vi "MS Auto Operation.vi"() -> ()   [LabVIEW 2016]
uses:
  <vilib>/Analysis/Matrix/Datatypes/RealMatrix.ctl
  Subsystems/Global Variables.vi
  <vilib>/FPGAPlugInAG/PXI-7833R/niLvFpga_Open_PXI-7833R.vi
  <vilib>/Utility/error.llb/Error Cluster From Error Code.vi
  <vilib>/rvi/errors/niLvFpgaAdjustHostInterfaceError.vi
  <vilib>/FPGAPlugInAG/PXI-7833R/niLvFpga_Reset_PXI-7833R.vi
  <vilib>/FPGAPlugInAG/PXI-7833R/niLvFpga_Close_PXI-7833R.vi
  <vilib>/rvi/interface/nirviOpenFPGA/nirviOpenFPGA.xnode
  FPGA Bitfiles/PhantomControlPI_FPGATarget_QuadCtr2_E2412E44.lvbitx
  IRISS_FPGA_IO.vi
  <vilib>/rvi/interface/nirviReadWriteControl/nirviReadWriteControl.xnode
  <vilib>/rvi/interface/nirviMethod/nirviMethod.xnode
  <vilib>/rvi/interface/nirviCloseFPGA/nirviCloseFPGA.xnode
  Library/KevinLibraryAll/labview2011/kevLib2011.lvlib
  <vilib>/Analysis/Matrix/NI_Matrix.lvlib
  NiFpgaLv.dll
panel:
  out "Online Eye Model":T1
  in  "To Regulation":bool
  out "Trajectory Cluster":T2
  out "Eye Model Cluster":T4={"X Grid"=[], "Y Grid"=[], "Za_true Surf"=[], "Iris Center"=[], "Zp_true Surf"=[], "Pinv"=[[1.0, 0.0], [0.0, 1.0]], "za_true"=5.0, "za_work"=1.0, "zp_work"=-1.0, "zp_true"=-5.0}
  out "Update Mdl & Traj":bool=TRUE
  in  "Initialize":bool caption="To M/S"
  out "Stage PID Cluster":T5={"Stage Z PID"={"Kp"=0.0005, "Kd"=0.001, "Ki"=0.0}, "Stage Y PID"={"Kp"=0.0003, "Kd"=0.01, "Ki"=0.0}, "Stage X PID"={"Kp"=0.0003, "Kd"=0.01, "Ki"=0.0}}
  out "L1 to L4 PID Cluster":T6={"L1 PID Gains"={"Kp"=0.005, "Kd"=0.5, "Ki"=0.0005}, "L2 PID Gains"={"Kp"=0.01, "Kd"=1.0, "Ki"=0.0005}, "L3 PID Gains"={"Kp"=0.05, "Kd"=1.0, "Ki"=0.0005}, "L4 PID Gains"={"Kp"=0.1, "Kd"=1.0, "Ki"=0.0005}}
  in  "IRISS GUI":T7(tab)
  in  "Reroute Hold [sec]":dbl=10.0 caption="Hold [sec]"
  out "X Stage out [mm] 2":dbl caption="Stage X [mm]" format="%#.4f"
  out "Z Stage out [mm] 2":dbl caption="Stage Z [mm]" format="%#.4f"
  out "Y Stage out [mm] 2":dbl caption="Stage Y [mm]" format="%#.4f"
  out "Vacuum Force [mmHg]  2":i32 caption="[mmHg]"
  out "Next Speed":dbl=0.8 format="%#.2gx"
  out "Current Speed":dbl=0.2 format="%#_2gx"
  out "Next Depth":dbl=40.0 format="%#_g%%"
  out "Current Depth":dbl=20.0 format="%#_6g%%"
  in  "Depth Offset":dbl min=-30.0 max=70.0 step=5.0 format="%#_g%%"
  in  "Refractice Index":dbl=1.35
  in  "PO No-Fly":dbl=5.0 step=0.1 format="%#.2g"
  out "PO Cruising":dbl=5.0 format="%#.2g"
  in  "Iris Center":dbl=5.0 step=0.1 format="%#.2g"
  in  "AN Cruising":dbl=5.0 step=0.1 format="%#.2g"
  in  "AN No-Fly":dbl=5.0 step=0.1 format="%#.2g"
  in  "Iris XY Scaling":dbl[](array[numeric])=[1.0, 1.0] caption="Iris Scaling" min=0.5 max=2.0 step=0.05
  in  "Iris XY Center":dbl[](array[numeric])=[0.0, 5.0] caption="Iris Center" min=-5.0 max=5.0 step=0.25
  out "Asgn Pt Out of Bound":bool caption="Assign Pt OOB"
  out "Finished Late Counts":u16
  out "Emergency alarm":bool
  out "Remote sender engaged":bool
  in  "L2 PID Gains":cluster{"Kp":dbl, "Kd":dbl, "Ki":dbl}={"Kp"=0.01, "Kd"=1.0, "Ki"=0.005}
  in  "L3 PID Gains":cluster{"Kp":dbl, "Kd":dbl, "Ki":dbl}={"Kp"=0.05, "Kd"=1.0, "Ki"=0.0005}
  in  "L4 PID Gains":cluster{"Kp":dbl, "Kd":dbl, "Ki":dbl}={"Kp"=0.1, "Kd"=0.1, "Ki"=0.0005}
  in  "L1 PID Gains":cluster{"Kp":dbl, "Kd":dbl, "Ki":dbl}={"Kp"=0.01, "Kd"=0.5, "Ki"=0.001}
  out "Current System State":T8(ring)
  out "State changing":bool
  out "Current Run No.":u8
  out "No. of Runs":i32=5
  out "Tip out Posit":dbl[](array[numeric]) caption="Position [mm]" format="%#.3f"
  out "Tip cmd Posit":dbl[](array[numeric]) caption="Command [mm]" format="%#.3f"
  out "L4 out Posit":dbl caption="y [deg]" format="%#.2g"
  out "L4 cmd Posit":dbl caption="r [deg]" format="%#.2g"
  out "L3 out Posit":dbl caption="y [mm]" format="%#.2g"
  out "L3 cmd Posit":dbl caption="r [mm]" format="%#.2g"
  out "L2 out Posit":dbl caption="y [deg]" format="%#.2g"
  out "L2 cmd Posit":dbl caption="r [deg]" format="%#.2g"
  out "L1 out Posit":dbl caption="y [deg]" format="%#.2g"
  out "L1 cmd Posit":dbl caption="r [deg]" format="%#.2g"
  out "State Flag Array":bool[](array[boolean])
  in  "Speed Override":u16(ring)=3 items=["4x", "3x", "2x", "1x", "0.5x", "0.2x", "0.1x", "PAUSE"]
  out "Timer":i32 format="%<%M:%S>t"
  in  "Assign Point [mm]":dbl[](array[numeric])=[0.0, 5.0, 0.0]
  in  "Go to Assign Pt":bool
  out "Irrigation Engaged? 2":bool caption="Irrigation Engaged"
  in  "Clear Charts":bool
  out "AC Pressure [mmHg]":sgl
  out "Elaspsed Time":sgl
  in  "File Path":path=path "C:/KevData1.txt"
  in  "Take IOP Data":bool
  out "IOP File Exists":bool
  in  "Seconds of Data":sgl=5.0
  out "Period [ms]":i64=10
  in  "Irrigation?":bool
  in  "PID ON/OFF":bool
  in  "Vac PID Gains":cluster{"Kp":dbl, "Kd":dbl, "Ki":dbl, "Ts":dbl}={"Kp"=5.0, "Kd"=0.0, "Ki"=5.0, "Ts"=0.01}
  in  "Vac Cmd":sgl min=0 max=100 step=1 format="%#_13g"
  in  "Target IOP":sgl=20.0 min=0 max=100 step=1 format="%#_13g"
  out "IOP Ctrl":T9(graph)
  out "Pressure Sensors":T10(graph)
  in  "Remote Control Source":u16(ring) caption="Remote Source" items=["Surgical Console", "Joystick"]
  in  "Reset Joystick":bool caption="Encoder Reset"
  in  "Robot Command":dbl[](array[numeric])=[0.0, 0.0, 0.0, 0.0]
  out "OCT Z out [mm]":dbl caption="OCT Out Z [mm]" format="%#.4f"
  out "OCT Z cmd [mm]":dbl=6.0 caption="OCT Z Ref [mm]" min=0.0 max=12.0 step=0.5
  in  "OCT Z PID Gains":cluster{"Kp":dbl, "Kd":dbl, "Ki":dbl}={"Kp"=0.0003, "Kd"=0.0001, "Ki"=0.01}
  out "Z Stage out [mm]":dbl caption="Output Z [mm]" format="%#.4f"
  out "Z Stage cmd [mm]":dbl=6.0 caption="Reference Z [mm]" min=0.0 max=12.0 step=0.5
  out "Y Stage out [mm]":dbl caption="Output Y [mm]" format="%#.4f"
  out "Y Stage cmd [mm]":dbl=6.0 caption="Reference Y  [mm]" min=0.0 max=12.0 step=0.5
  out "X Stage out [mm]":dbl caption="Output X [mm]" format="%#.4f"
  out "X Stage cmd [mm]":dbl=6.0 caption="Reference X [mm]" min=0.0 max=12.0 step=0.5
  in  "Stage Z PID Gains":cluster{"Kp":dbl, "Kd":dbl, "Ki":dbl}={"Kp"=0.0005, "Kd"=0.001, "Ki"=0.0}
  in  "Stage Y PID Gains":cluster{"Kp":dbl, "Kd":dbl, "Ki":dbl}={"Kp"=0.0001, "Kd"=0.005, "Ki"=0.0}
  in  "Stage X PID Gains":cluster{"Kp":dbl, "Kd":dbl, "Ki":dbl}={"Kp"=0.0003, "Kd"=0.01, "Ki"=0.0}
  in  "Reroute Transit Vacf":dbl=100.0
  out "Irrigation Engaged?":bool
  in  "Z Rot Axis":dbl=1.0
  in  "Z Dist Thld":dbl[](array[numeric])=[0.5, 2.0] caption="Z Distance Threshould"
  in  "Vac Extremum":dbl[](array[numeric])=[80.0, 100.0] caption="Vacuum Extremum"
  out "Accurus Button":bool[](array[boolean]) caption="Remote Button Command"
  in  "Max Limit [mmHg]":dbl=600.0
  in  "Control: Vacuum Force":i8(slide) min=0 max=78 step=1 scale=0.0..78.0
  out "Voltage Output Ch. B":dbl(graph)
  out "Voltage Output Ch. A":dbl(graph)
  out "Accurus Engaged?":bool
  out "Vacuum Force [mmHg]":i32
  in  "Stop-and-Go":bool=TRUE
  in  "Min PC Gap":dbl=0.1 caption="Min PC Gap [mm]" min=0.0 max=10.0 step=0.1 format="%#.3g"
  in  "Min AC Gap":dbl=0.1 caption="Min AC Gap [mm]" min=0.0 max=10.0 step=0.1 format="%#.3g"
  out "Scaling":dbl[](array[numeric])=[1.0, 1.0, 1.0] caption="S" min=0.5 max=1.5 step=0.05 format="%#_3g"
  in  "Joint Limits":dbl[][](array[numeric])=[[-8.0, 35.0], [-35.0, 35.0], [-5.0, 10.0], [-180.0, 180.0]] format="%#.3g"
  out "First Trk Pt":dbl[](array[numeric]) format="%#.3g"
  in  "Offset Home 2 RCM":dbl[](array[numeric])=[-7.7, 37.0, 55.0, 0.0] format="%#.3g"
  out "Error(s) Out on Program End":errorcluster
  out "L4 Waveform Graph":dbl[](graph)
  out "L3 Waveform Graph":dbl[](graph)
  out "L2 Waveform Graph":dbl[](graph)
  out "L1 Waveform Graph":dbl[](graph)
  in  "Aiming Pt":dbl[](array[numeric])=[10.0, 0.0, -1.0, 0.0] format="%#.3g"
  in  "Engage Pt":dbl[](array[numeric])=[15.0, 0.0, 3.0, 0.0] format="%#.3g"
  in  "Rotation":dbl[](array[numeric])=[0.0, 0.0, 0.0] caption="R [deg]" min=-15.0 max=15.0 step=0.5 format="%#_3g"
  out "Translation":dbl[](array[numeric]) caption="T [mm]" min=-3.0 max=3.0 step=0.1 format="%#_3g"
  in  "Inc Ctrl":dbl[](array[numeric])=[0.1, 0.05, 0.05] caption="Increment Control"
  in  "Load Traj":bool caption="To M/S"
  in  "MS/Auto":bool
  in  "Retract":bool caption="To M/S"
  in  "Stop Accurus":bool caption="To M/S"
  in  "L3 Go Home":bool caption="To M/S"
  in  "Track":bool caption="To M/S"
  in  "Insert":bool caption="To M/S"
  in  "Program Stop":bool
  # "M/S\n\nAuto"
  # "Robot Status"
  # "Tool Tip Location"
  # "Tracking Planning"
  # "L1"
  # "X\nY\nZ"
  # "X\nY\nZ"
  # "L2"
  # "System Progress"
  # "Assign Point Rerouting"
  # "X\nY\nZ"
  # "L3"
  # "Homing finished"
  # "M/S initialization finished"
  # "Tool Cruising Boundaries"
  # "Trajecoty loading finished"
  # "XY-plane"
  # "Z-axis"
  # "Aiming finished"
  # "L4"
  # "Tool engaged"
  # "Tracking initialization finished"
  # "In Tracking"
  # "Rerouting finished"
  # "In regulation"
  # "Vacuum"
  # "X\nY"
  # "X\nY"
  # "L1"
  # "L2"
  # "L3"
  # "L4"
  # "Data Saving"
  # "IOP Feedback Control"
  # "XYZ Stage Control"
  # "OCT Z-Axis"
  # "Foot Pedal Buttons"
  # "Irrigation and Aspiration"
  # "Button 1"
  # "Button 2"
  # "Button 3"
  # "Rotation & Vacuum Force Scheduling"
  # "Joint Motion & Control"
  # "Calibration"
  # "Space Deform Parameters"
  # "L1"
  # "[deg]"
  # "S"
  # "L2"
  # "[deg]"
  # "R"
  # "[deg]"
  # "L3"
  # "[mm]"
  # "T"
  # "[mm]"
  # "L4"
  # "[deg]"
  # "First Track Point"
  # "AC & PC Gap"
  # "L1"
  # "[deg]"
  # "L2"
  # "[deg]"
  # "L3"
  # "[mm]"
  # "L4"
  # "[deg]"
  # "Error Message"
  # "Tracking Joint Limits"
  # "Incision"
  # "Min."
  # "Max."
  # "L1"
  # "L1"
  # "[deg]"
  # "L2"
  # "L2"
  # "[deg]"
  # "L3"
  # "L3"
  # "[mm]"
  # "L4"
  # "L4"
  # "[deg]"
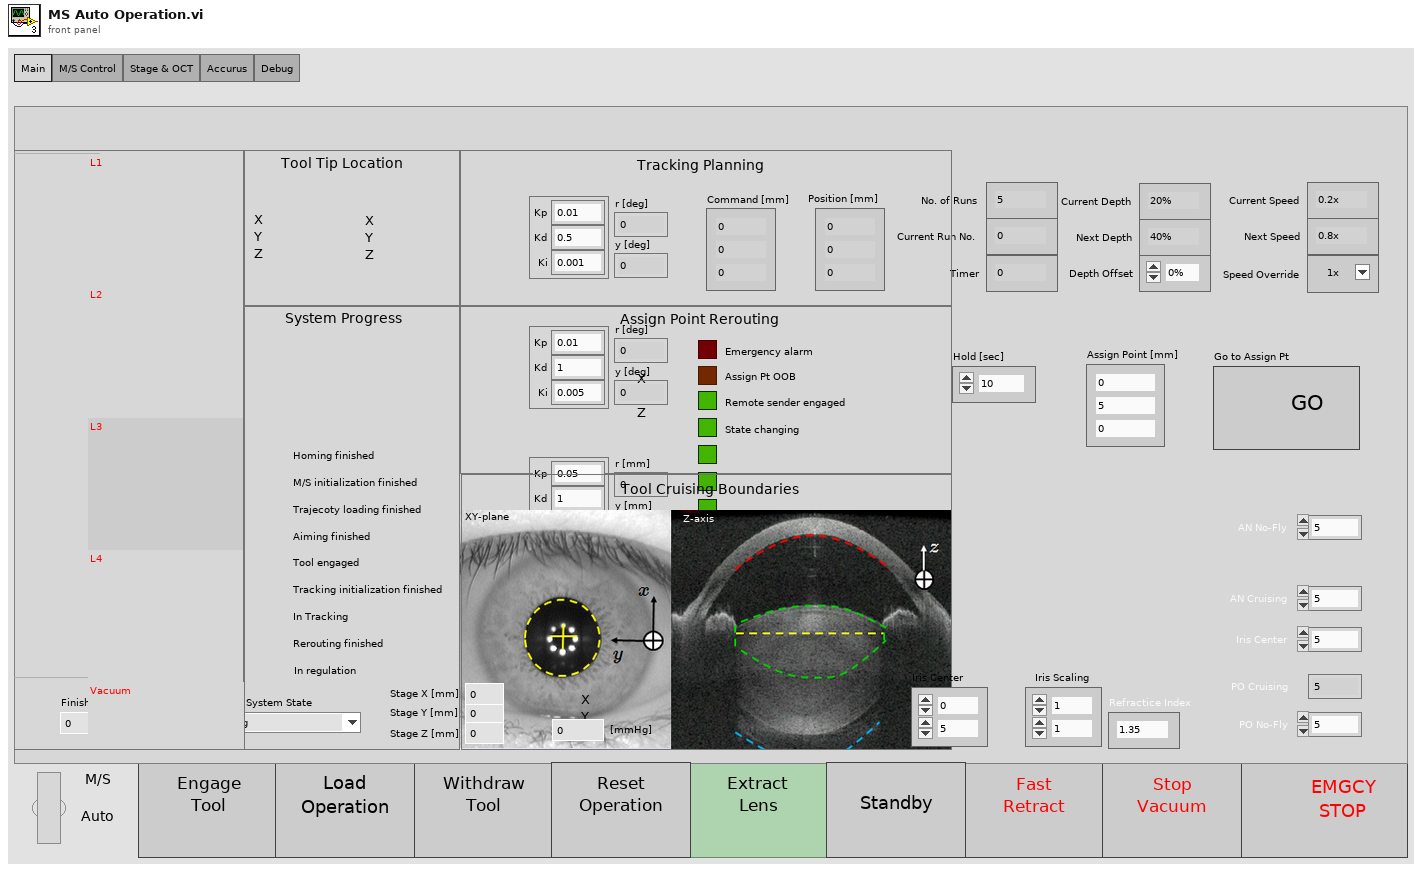
[diagram p1: front panel]
types:
  T1 = cluster{"za_true":dbl, "za_work":dbl, "zi":dbl, "zp_work":dbl, "zp_true":dbl, "Iris XY Center":dbl[], "Iris XY Scaling":dbl[]}
  T2 = cluster{"Traj Px Array":dbl[], "Traj Py Array":dbl[], "Traj Pz Array":dbl[], "Speed Array":dbl[], "Depth Array":dbl[]}
  T3 = typedef "NI_Matrix.lvlib/RealMatrix.ctl" = dbl[][]
  T4 = cluster{"X Grid":dbl[], "Y Grid":dbl[], "Za_true Surf":dbl[][], "Iris Center":dbl[], "Zp_true Surf":dbl[][], "Pinv":T3, "za_true":dbl, "za_work":dbl, "zp_work":dbl, "zp_true":dbl}
  T5 = cluster{"Stage Z PID":cluster{"Kp":dbl, "Kd":dbl, "Ki":dbl}, "Stage Y PID":cluster{"Kp":dbl, "Kd":dbl, "Ki":dbl}, "Stage X PID":cluster{"Kp":dbl, "Kd":dbl, "Ki":dbl}}
  T6 = cluster{"L1 PID Gains":cluster{"Kp":dbl, "Kd":dbl, "Ki":dbl}, "L2 PID Gains":cluster{"Kp":dbl, "Kd":dbl, "Ki":dbl}, "L3 PID Gains":cluster{"Kp":dbl, "Kd":dbl, "Ki":dbl}, "L4 PID Gains":cluster{"Kp":dbl, "Kd":dbl, "Ki":dbl}}
  T7 = enum32{"Main", "M/S Control", "Stage & OCT", "Accurus", "Debug"}
  T8 = enum16{"Homing", "M/S Initialization", "M/S Operation", "Aiming", "Engaging", "Trajectory Loading", "Tracking Initialization", "Tracking", "Rerouting", "Regulation"}
  T9 = cluster{"[0]":sgl, "[1]":sgl, "[2]":sgl, "[3]":sgl, "[4]":sgl, "[5]":sgl, "[6]":sgl, "[7]":sgl, "[8]":sgl}
  T10 = cluster{"pressure sensors[0]":sgl, "pressure sensors[1]":sgl, "pressure sensors[2]":sgl, "pressure sensors[3]":sgl, "pressure sensors[4]":sgl, "pressure sensors[5]":sgl, "pressure sensors[6]":sgl, "pressure sensors[7]":sgl, "pressure sensors[8]":sgl}
  T11 = cluster{"Prev L1 to L4 Posit":dbl[], "Prev Stage Posit":dbl[], "Prev OCT Z Posit":dbl}
  T12 = cluster{"L1 to L4 PID Cluster":cluster{"L1 PID Gains":cluster{"Kp":dbl, "Kd":dbl, "Ki":dbl}, "L2 PID Gains":cluster{"Kp":dbl, "Kd":dbl, "Ki":dbl}, "L3 PID Gains":cluster{"Kp":dbl, "Kd":dbl, "Ki":dbl}, "L4 PID Gains":cluster{"Kp":dbl, "Kd":dbl, "Ki":dbl}}, "Stage PID Cluster":cluster{"Stage Z PID":cluster{"Kp":dbl, "Kd":dbl, "Ki":dbl}, "Stage Y PID":cluster{"Kp":dbl, "Kd":dbl, "Ki":dbl}, "Stage X PID":cluster{"Kp":dbl, "Kd":dbl, "Ki":dbl}}, "OCT Z PID Gains":cluster{"Kp":dbl, "Kd":dbl, "Ki":dbl}}
  T13 = enum8{"Enabled", "Disabled", "Disabled and Grayed Out"}
  T14 = cluster{"Last L1 to L4 Posit":dbl[], "Last Stage Posit":dbl[], "Last OCT Z Posit":dbl}
  T15 = cluster{"za_true_0":dbl, "za_work_0":dbl, "zp_work_0":dbl, "zp_true_0":dbl, "IrisCenter_0":dbl[]}
  T16 = cluster{"X Grid":dbl[], "Y Grid":dbl[], "Za_true Surf":dbl[][], "Iris Center":dbl[], "Zp_true Surf":dbl[][], "Real Matrix":T3, "za_true":dbl, "za_work":dbl, "zp_work":dbl, "zp_true":dbl}
  T17 = cluster{"Accurus button":bool[], "Accurus engaged?":bool, "Vacuum Force":i32, "Accurus Ch. A Vout":dbl, "Accurus Ch. B Vout":dbl, "Irrigation engaged?":bool}
  T18 = cluster{"pressure sensors[0]":sgl, "pressure sensors[1]":sgl, "pressure sensors[2]":sgl, "pressure sensors[3]":sgl, "pressure sensors[4]":sgl, "pressure sensors[5]":sgl, "pressure sensors[6]":sgl, "pressure sensors[7]":sgl, "pressure sensors[8]":sgl}[]
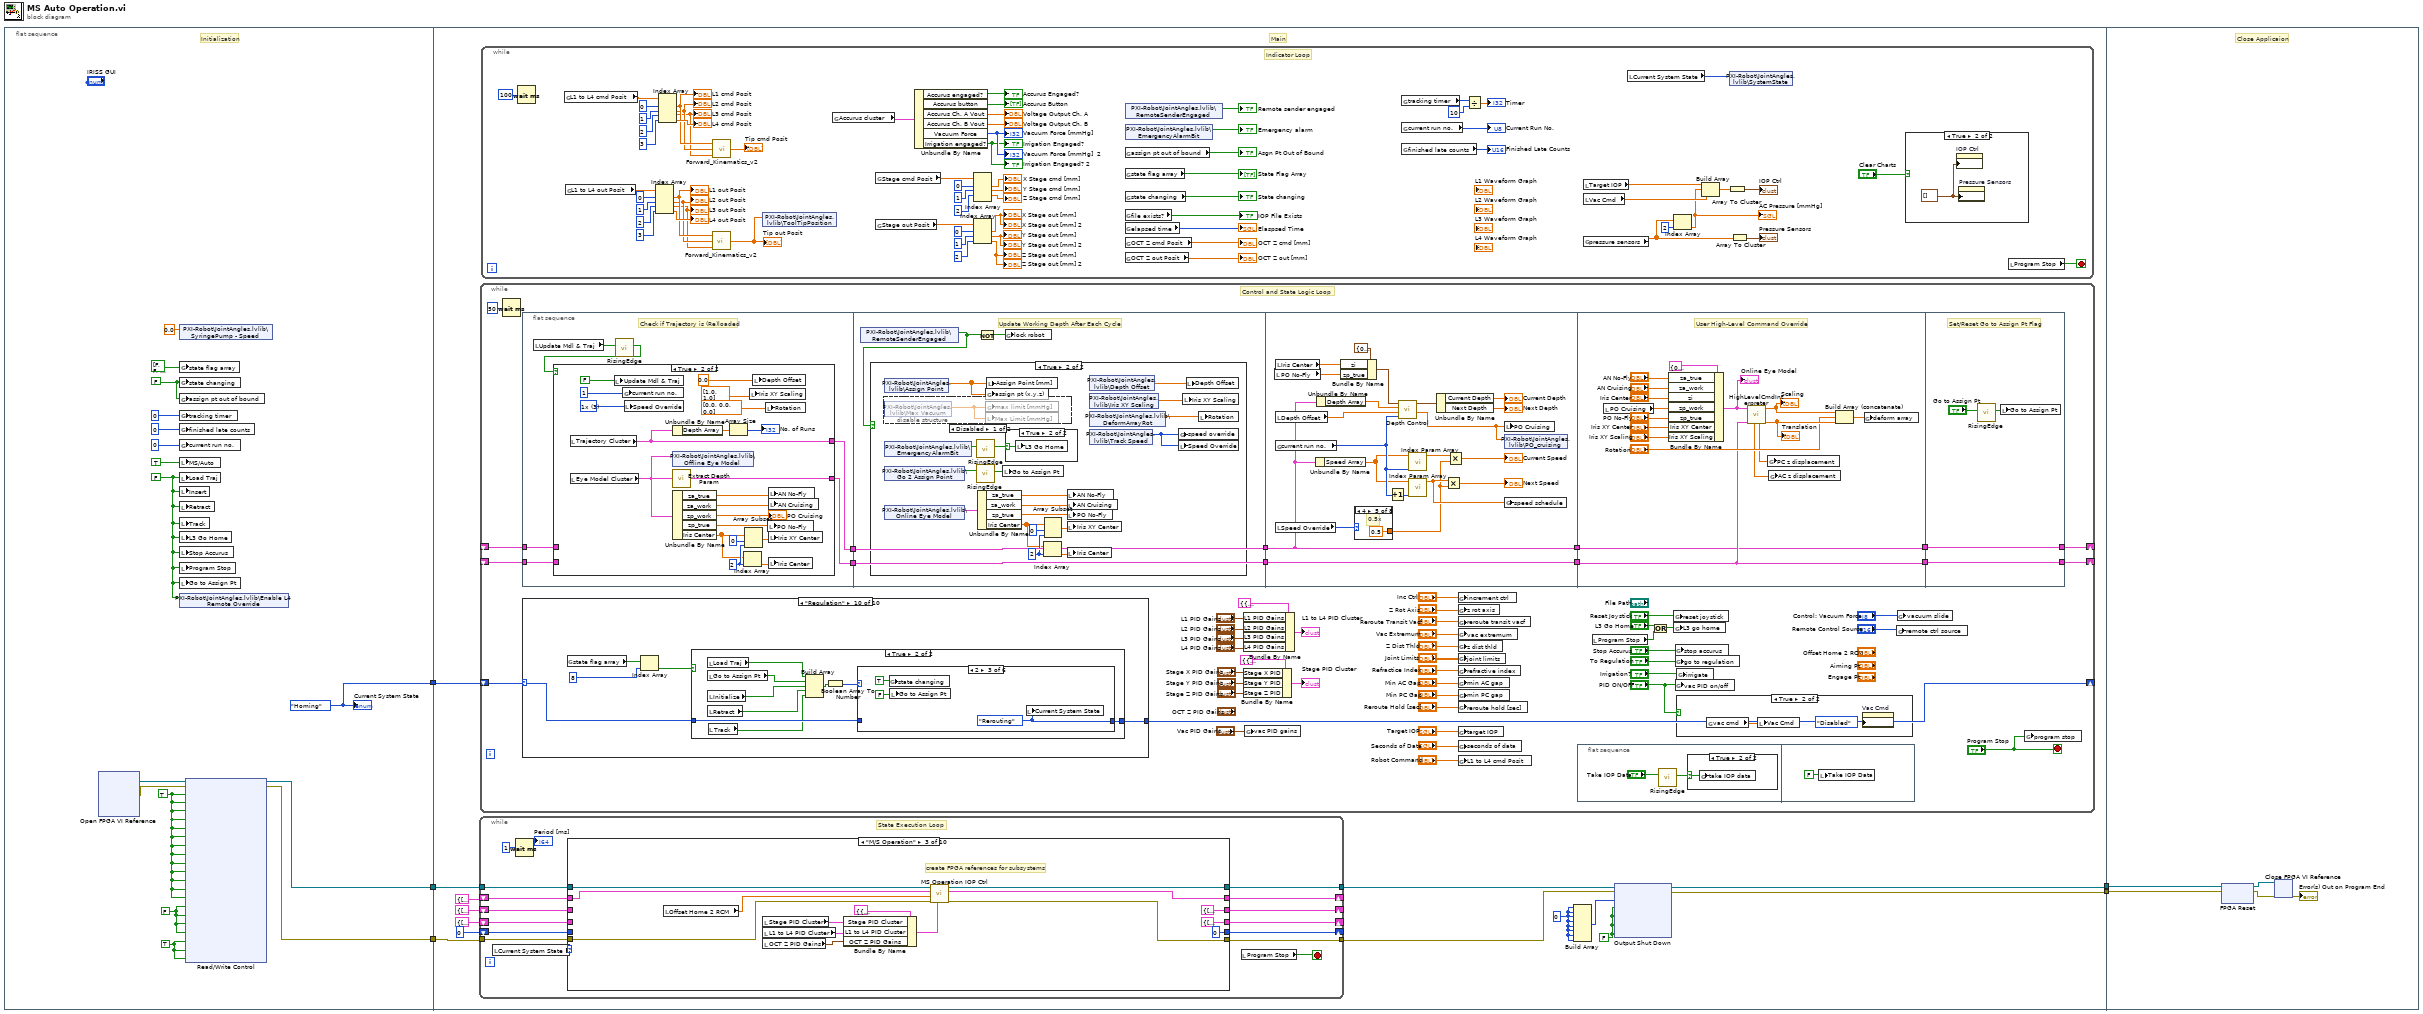
[diagram p0: block diagram]
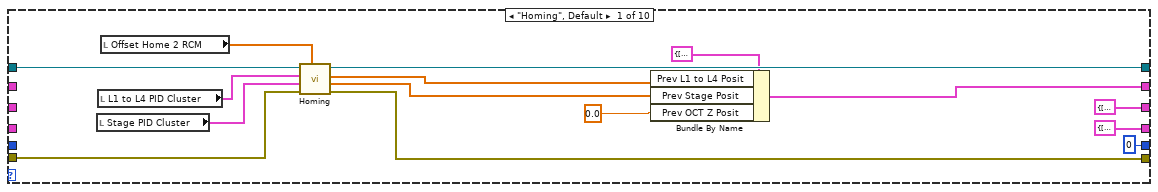
[diagram p3: hidden frame]
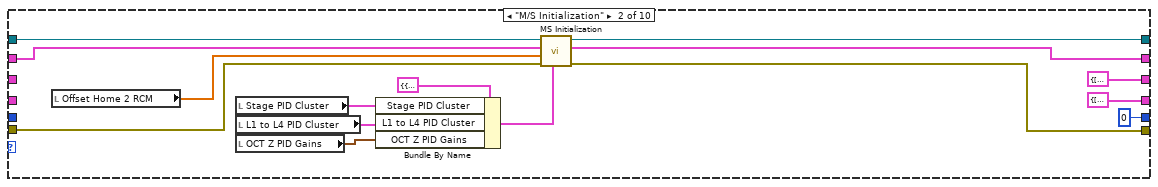
[diagram p4: hidden frame]
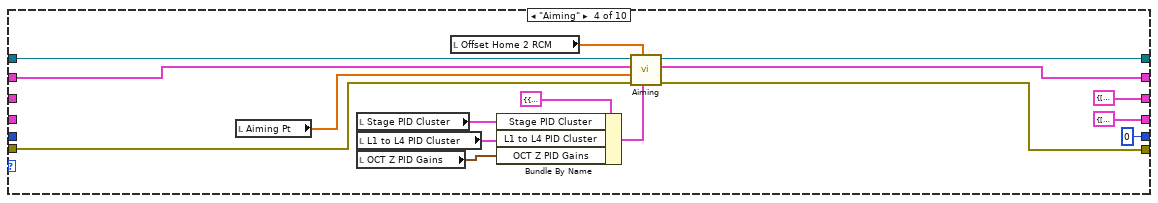
[diagram p5: hidden frame]
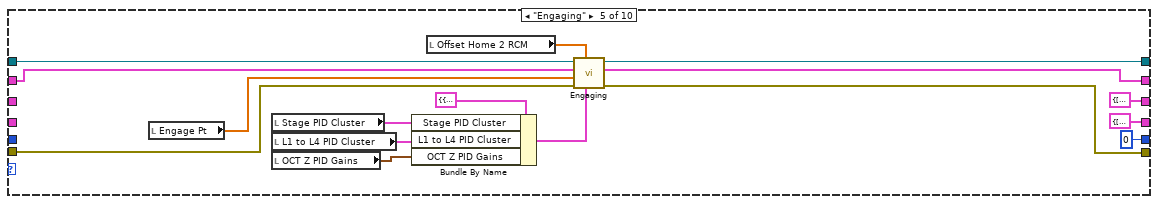
[diagram p6: hidden frame]
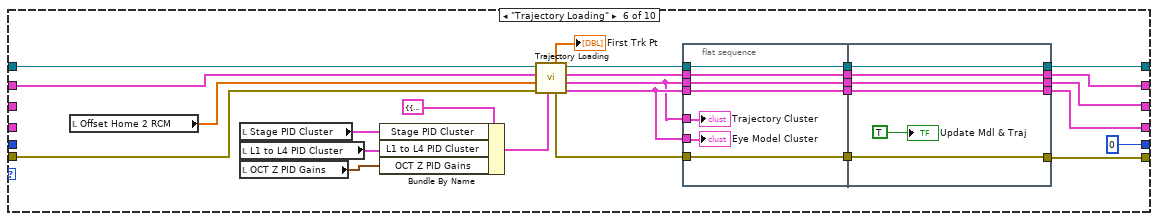
[diagram p7: hidden frame]
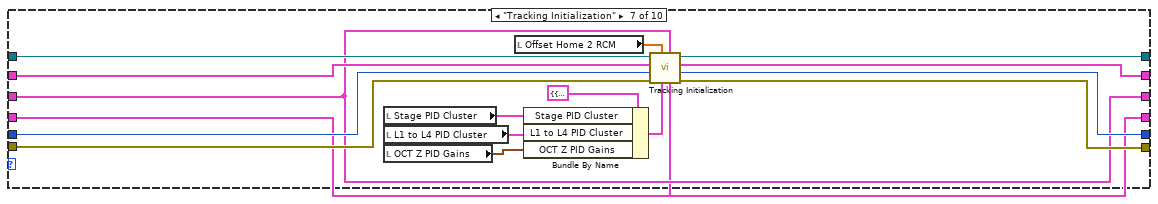
[diagram p8: hidden frame]
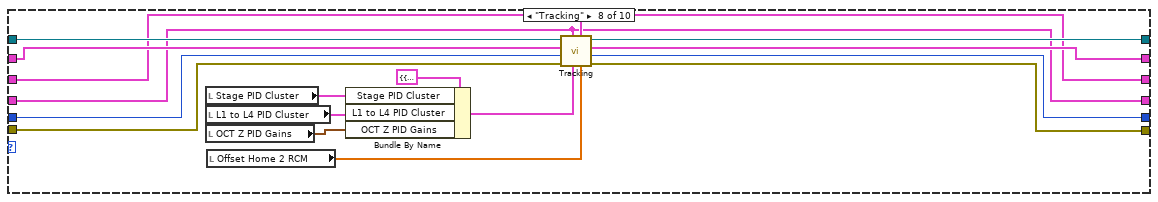
[diagram p9: hidden frame]
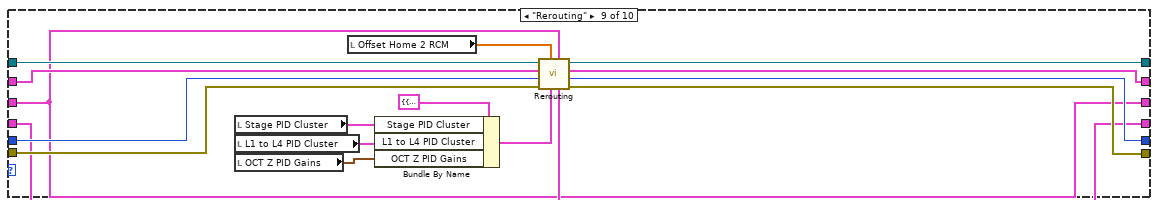
[diagram p10: hidden frame]
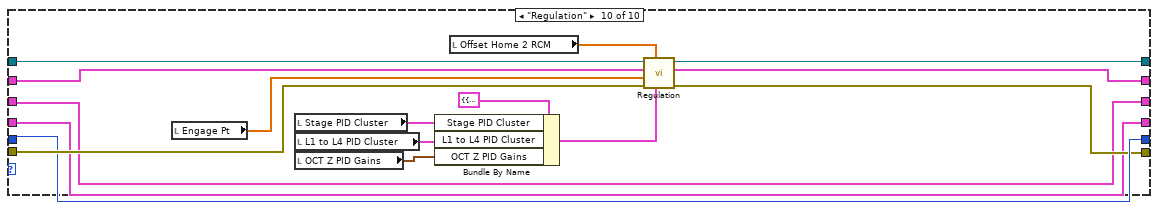
[diagram p11: hidden frame]
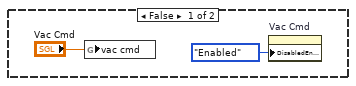
[diagram p13: hidden frame]
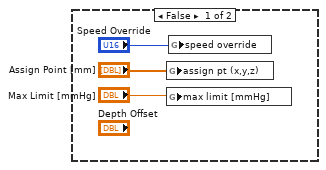
[diagram p15: hidden frame]
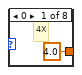
[diagram p18: hidden frame]
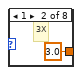
[diagram p19: hidden frame]
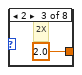
[diagram p20: hidden frame]
diagram:
  n1 = flat-sequence {
    tunnel: [w16] -> w5
    tunnel: [w15] -> w4
    tunnel: [w10] -> w3
    tunnel: w5 -> [w34]
    tunnel: w4 -> [w35]
    tunnel: w3 -> [w26]
    tunnel: [w28] -> w2
    tunnel: [w27] -> w1
    tunnel: w2 -> [w695]
    tunnel: w1 -> [w696]
    frame #0 {
      w10 = T8."Homing" ("Current State")
      w12 = FALSE ("state changing")
      w20 = TRUE ("Conn0/DIO12 Button 1")
      w19 = FALSE ("Reset")
      w21 = TRUE ("Reset")
      w13 = FALSE ("program stop")
      # "Initialization"
      n2 = xnode "Open FPGA VI Reference"() -> ("FPGA VI Reference Out"=w18:refnum<k20>, "error out"=w17:errorcluster)  [unwired: 2 in]
      n3 = shared-variable "PXI-Robot\\JointAngles.lvlib\\SyringePump - Speed"(0.0 ("SyringePump - Speed")) -> ()  [unwired: 1 in, 1 out]
      n4 = global write "Global Variables.vi" "state flag array"(bool[] [FALSE, FALSE, FALSE, FALSE, FALSE, FALSE, FALSE, FALSE, FALSE] ("state flag array")) -> ()
      n5 = global write "Global Variables.vi" "state changing"(w12) -> ()
      n6 = global write "Global Variables.vi" "assign pt out of bound"(w12) -> ()
      n7 = global write "Global Variables.vi" "tracking timer"(0 ("finished late counts")) -> ()
      n8 = global write "Global Variables.vi" "finished late counts"(u16 0 ("finished late counts")) -> ()
      n9 = global write "Global Variables.vi" "current run no."(u8 0 ("current run no.")) -> ()
      n10 = local write "MS/Auto"(TRUE ("MS/Auto")) -> ()
      n11 = local write "Load Traj"(w13) -> ()
      n12 = local write "Insert"(w13) -> ()
      n13 = local write "Retract"(w13) -> ()
      n14 = local write "Track"(w13) -> ()
      n15 = local write "L3 Go Home"(w13) -> ()
      n16 = local write "Stop Accurus"(w13) -> ()
      n17 = local write "Program Stop"(w13) -> ()
      n18 = local write "Go to Assign Pt"(w13) -> ()
      n19 = shared-variable "PXI-Robot\\JointAngles.lvlib\\Enable L4 Remote Override"(w13) -> ()  [unwired: 1 in, 1 out]
      n20 = xnode "Read/Write Control"("FPGA VI Reference In"=w18, "error in"=w17, "Reset 1"=w21, "Reset 3"=w21, "Reset 9"=w21, "Reset 10"=w21, "Reset 11"=w21, "Reset 12"=w21, "Reset 13"=w21, "Reset 14"=w21, "Reset 15"=w21, "Reset 16"=w21, "Reset 17"=w21, "Reset C1-1"=w21, "Reset C1-4"=w21, "INHB X"=w19, "INHB Y"=w19, "INHB Z"=w19, "INHB OCT Mot"=w19, "Conn0/DIO12 Button 1"=w20, "Conn0/DIO13 Button 2"=w20, "Conn0/DIO15 Button 4"=w20) -> ("FPGA VI Reference Out"=w15:refnum<k20>, "error out"=w16:errorcluster)
      "Current System State" <- w10
    }
    frame #1 {
      w32 = FALSE
      w24 = i16 0 ("element")
      # "Main"
      n21 = while {
        tunnel: w35 -> [w116]
        tunnel: w34 -> [w115]
        tunnel: [w114] -> w30
        tunnel: [w113] -> w29
        shift-right: [w111] -> _
        shift-left: T11 {"Prev L1 to L4 Posit"=[0.0, 0.0, 0.0, 0.0], "Prev Stage Posit"=[6.0, 6.0, 6.0], "Prev OCT Z Posit"=0.0} ("Prev Posit Cluster") -> [w112]
        shift-right: [w109] -> _
        shift-left: 0 -> [w108]
        shift-right: [w107] -> _
        shift-left: T2 {"Traj Px Array"=[], "Traj Py Array"=[], "Traj Pz Array"=[], "Speed Array"=[], "Depth Array"=[]} ("Trajectory Cluster") -> [w105]
        shift-right: [w106] -> _
        shift-left: T4 {"X Grid"=[], "Y Grid"=[], "Za_true Surf"=[], "Iris Center"=[0.0, 5.0, 0.0], "Zp_true Surf"=[], "Pinv"=[[1.0, 0.0], [0.0, 1.0]], "za_true"=0.0, "za_work"=0.0, "zp_work"=0.0, "zp_true"=0.0} ("Eye Model Cluster") -> [w104]
        stop <- w110 stop-if-true
        # "State Execution Loop"
        n22 = local read "Current System State"() -> (w117:T8)
        n23 = Wait (ms)(milliseconds to wait=u32 1) -> ()  [unwired: 1 out]
        n24 = case shown="\"M/S Operation\"" w117 {
          tunnel: w116 -> [w133 w148 w163 w177 w194 w221 w250 w266 w281 w293]
          tunnel: w115 -> [w132 w147 w162 w168 w186 w220 w249 w265 w275 w290]
          tunnel: [w131 w146 w161 w174 w195 w202 w248 w264 w282 w287] -> w114
          tunnel: [w130 w145 w160 w178 w183 w208 w247 w263 w269 w285] -> w113
          tunnel: w112 -> [_ w144 w159 w175 w184 w219 w245 w262 w274 w292]
          tunnel: [w129 w143 w158 w179 w192 w207 w246 w261 w272 w286] -> w111
          tunnel: [0 ("Last Index") 0 ("Last Index") 0 ("Last Index") 0 ("Last Index") 0 ("Last Index") 0 w237 w251 w270 w288] -> w109
          tunnel: w108 -> [_ _ _ _ _ _ w238 w252 w271 w288]
          tunnel: [T2 {"Traj Px Array"=[], "Traj Py Array"=[], "Traj Pz Array"=[], "Speed Array"=[], "Depth Array"=[]} ("Trajectory Cluster") T2 {"Traj Px Array"=[], "Traj Py Array"=[], "Traj Pz Array"=[], "Speed Array"=[], "Depth Array"=[]} ("Trajectory Cluster") T2 {"Traj Px Array"=[], "Traj Py Array"=[], "Traj Pz Array"=[], "Speed Array"=[], "Depth Array"=[]} ("Trajectory Cluster") T2 {"Traj Px Array"=[], "Traj Py Array"=[], "Traj Pz Array"=[], "Speed Array"=[], "Depth Array"=[]} ("Trajectory Cluster") T2 {"Traj Px Array"=[], "Traj Py Array"=[], "Traj Pz Array"=[], "Speed Array"=[], "Depth Array"=[]} ("Trajectory Cluster") w198 w236 w255 w267 w284] -> w107
          tunnel: [T4 {"X Grid"=[], "Y Grid"=[], "Za_true Surf"=[], "Iris Center"=[0.0, 5.0, 0.0], "Zp_true Surf"=[], "Pinv"=[[1.0, 0.0], [0.0, 1.0]], "za_true"=0.0, "za_work"=0.0, "zp_work"=0.0, "zp_true"=0.0} ("Eye Model Cluster") T4 {"X Grid"=[], "Y Grid"=[], "Za_true Surf"=[], "Iris Center"=[0.0, 5.0, 0.0], "Zp_true Surf"=[], "Pinv"=[[1.0, 0.0], [0.0, 1.0]], "za_true"=0.0, "za_work"=0.0, "zp_work"=0.0, "zp_true"=0.0} ("Eye Model Cluster") T4 {"X Grid"=[], "Y Grid"=[], "Za_true Surf"=[], "Iris Center"=[0.0, 5.0, 0.0], "Zp_true Surf"=[], "Pinv"=[[1.0, 0.0], [0.0, 1.0]], "za_true"=0.0, "za_work"=0.0, "zp_work"=0.0, "zp_true"=0.0} ("Eye Model Cluster") T4 {"X Grid"=[], "Y Grid"=[], "Za_true Surf"=[], "Iris Center"=[0.0, 5.0, 0.0], "Zp_true Surf"=[], "Pinv"=[[1.0, 0.0], [0.0, 1.0]], "za_true"=0.0, "za_work"=0.0, "zp_work"=0.0, "zp_true"=0.0} ("Eye Model Cluster") T4 {"X Grid"=[], "Y Grid"=[], "Za_true Surf"=[], "Iris Center"=[0.0, 5.0, 0.0], "Zp_true Surf"=[], "Pinv"=[[1.0, 0.0], [0.0, 1.0]], "za_true"=0.0, "za_work"=0.0, "zp_work"=0.0, "zp_true"=0.0} ("Eye Model Cluster") w197 w235 w254 w268 w283] -> w106
          tunnel: w105 -> [_ _ _ _ _ _ w236 w255 w267 w284]
          tunnel: w104 -> [_ _ _ _ _ _ w235 w254 w268 w283]
          frame "Homing", Default {
            n25 = local read "Stage PID Cluster"() -> (w125:T5)
            n26 = local read "L1 to L4 PID Cluster"() -> (w126:T6)
            n27 = local read "Offset Home 2 RCM"() -> (w128:dbl[])
            n28 = call "Homing.vi"("Offset Home 2 RCM"=w128, "error in"=w132, "Stage PID Cluster"=w125, "L1 to L4 PID Cluster"=w126, "FPGA VI Reference In"=w133) -> ("error out"=w130:errorcluster, "Last Stage Posit"=w122:dbl[], "Last L1 to L4 Posit"=w123:dbl[], "FPGA VI Reference Out"=w131:refnum<k20>)  [unwired: 3 in]
            n29 = Bundle By Name(cluster=T11 {"Prev L1 to L4 Posit"=[-0.5409, 0.04404050915429177, -1.917656453185038, 0.02068014705882353], "Prev Stage Posit"=[6.001471972029684, 5.996134588585126, 6.000298217087839], "Prev OCT Z Posit"=-0.0} ("Prev Posit Cluster"), "Prev L1 to L4 Posit"=w123, "Prev Stage Posit"=w122, "Prev OCT Z Posit"=0.0) -> (w129:T11)
          }
          frame "M/S Initialization" {
            n30 = local read "Offset Home 2 RCM"() -> (w137:dbl[])
            n31 = local read "Stage PID Cluster"() -> (w142:T5)
            n32 = local read "L1 to L4 PID Cluster"() -> (w141:T6)
            n33 = local read "OCT Z PID Gains"() -> (w140:cluster{"Kp":dbl, "Kd":dbl, "Ki":dbl})
            n34 = Bundle By Name(cluster=T12 {"L1 to L4 PID Cluster"={"L1 PID Gains"={"Kp"=0.005, "Kd"=0.5, "Ki"=0.0005}, "L2 PID Gains"={"Kp"=0.01, "Kd"=1.0, "Ki"=0.005}, "L3 PID Gains"={"Kp"=0.05, "Kd"=1.0, "Ki"=0.0005}, "L4 PID Gains"={"Kp"=0.1, "Kd"=0.1, "Ki"=0.0005}}, "Stage PID Cluster"={"Stage Z PID"={"Kp"=0.0005, "Kd"=0.001, "Ki"=0.0}, "Stage Y PID"={"Kp"=0.0003, "Kd"=0.01, "Ki"=0.0}, "Stage X PID"={"Kp"=0.0003, "Kd"=0.01, "Ki"=0.0}}, "OCT Z PID Gains"={"Kp"=0.0003, "Kd"=0.0001, "Ki"=0.01}} ("PID Cluster"), "Stage PID Cluster"=w142, "L1 to L4 PID Cluster"=w141, "OCT Z PID Gains"=w140) -> (w138:T12)
            n35 = call "MS Initialization.vi"("PID Cluster"=w138, "error in"=w147, "Offset Home 2 RCM"=w137, "Prev Posit Cluster"=w144, "FPGA VI Reference In"=w148) -> ("error out"=w145:errorcluster, "Last Posit Cluster"=w143:T14, "FPGA VI Reference Out"=w146:refnum<k20>)  [unwired: 4 in]
          }
          frame "M/S Operation" {
            # "create FPGA references for subsystems"
            n36 = local read "Offset Home 2 RCM"() -> (w152:dbl[])
            n37 = local read "Stage PID Cluster"() -> (w157:T5)
            n38 = local read "L1 to L4 PID Cluster"() -> (w156:T6)
            n39 = local read "OCT Z PID Gains"() -> (w155:cluster{"Kp":dbl, "Kd":dbl, "Ki":dbl})
            n40 = Bundle By Name(cluster=T12 {"L1 to L4 PID Cluster"={"L1 PID Gains"={"Kp"=0.005, "Kd"=0.5, "Ki"=0.0005}, "L2 PID Gains"={"Kp"=0.01, "Kd"=1.0, "Ki"=0.005}, "L3 PID Gains"={"Kp"=0.05, "Kd"=1.0, "Ki"=0.0005}, "L4 PID Gains"={"Kp"=0.1, "Kd"=0.1, "Ki"=0.0005}}, "Stage PID Cluster"={"Stage Z PID"={"Kp"=0.0005, "Kd"=0.001, "Ki"=0.0}, "Stage Y PID"={"Kp"=0.0003, "Kd"=0.01, "Ki"=0.0}, "Stage X PID"={"Kp"=0.0003, "Kd"=0.01, "Ki"=0.0}}, "OCT Z PID Gains"={"Kp"=0.0003, "Kd"=0.0001, "Ki"=0.01}} ("PID Cluster"), "Stage PID Cluster"=w157, "L1 to L4 PID Cluster"=w156, "OCT Z PID Gains"=w155) -> (w153:T12)
            n41 = call "MS Operation IOP Ctrl.vi"("PID Cluster"=w153, "error in"=w162, "Offset Home 2 RCM"=w152, "Prev Posit Cluster"=w159, "FPGA VI Reference In"=w163) -> ("error out"=w160:errorcluster, "Last Posit Cluster"=w158:T14, "FPGA VI Reference Out"=w161:refnum<k20>)  [unwired: 4 in]
          }
          frame "Aiming" {
            n42 = local read "Aiming Pt"() -> (w173:dbl[])
            n43 = local read "Stage PID Cluster"() -> (w172:T5)
            n44 = local read "L1 to L4 PID Cluster"() -> (w171:T6)
            n45 = local read "OCT Z PID Gains"() -> (w169:cluster{"Kp":dbl, "Kd":dbl, "Ki":dbl})
            n46 = local read "Offset Home 2 RCM"() -> (w176:dbl[])
            n47 = Bundle By Name(cluster=T12 {"L1 to L4 PID Cluster"={"L1 PID Gains"={"Kp"=0.005, "Kd"=0.5, "Ki"=0.0005}, "L2 PID Gains"={"Kp"=0.01, "Kd"=1.0, "Ki"=0.005}, "L3 PID Gains"={"Kp"=0.05, "Kd"=1.0, "Ki"=0.0005}, "L4 PID Gains"={"Kp"=0.1, "Kd"=0.1, "Ki"=0.0005}}, "Stage PID Cluster"={"Stage Z PID"={"Kp"=0.0005, "Kd"=0.001, "Ki"=0.0}, "Stage Y PID"={"Kp"=0.0003, "Kd"=0.01, "Ki"=0.0}, "Stage X PID"={"Kp"=0.0003, "Kd"=0.01, "Ki"=0.0}}, "OCT Z PID Gains"={"Kp"=0.0003, "Kd"=0.0001, "Ki"=0.01}} ("PID Cluster"), "Stage PID Cluster"=w172, "L1 to L4 PID Cluster"=w171, "OCT Z PID Gains"=w169) -> (w167:T12)
            n48 = call "Aiming.vi"("PID Cluster"=w167, "Offset Home 2 RCM"=w176, "error in"=w168, "Aiming Pt"=w173, "Prev Posit Cluster"=w175, "FPGA VI Reference In"=w177) -> ("error out"=w178:errorcluster, "Last Posit Cluster"=w179:T14, "FPGA VI Reference Out"=w174:refnum<k20>)  [unwired: 3 in]
          }
          frame "Engaging" {
            n49 = local read "Engage Pt"() -> (w185:dbl[])
            n50 = local read "Stage PID Cluster"() -> (w190:T5)
            n51 = local read "L1 to L4 PID Cluster"() -> (w189:T6)
            n52 = local read "OCT Z PID Gains"() -> (w188:cluster{"Kp":dbl, "Kd":dbl, "Ki":dbl})
            n53 = Bundle By Name(cluster=T12 {"L1 to L4 PID Cluster"={"L1 PID Gains"={"Kp"=0.005, "Kd"=0.5, "Ki"=0.0005}, "L2 PID Gains"={"Kp"=0.01, "Kd"=1.0, "Ki"=0.005}, "L3 PID Gains"={"Kp"=0.05, "Kd"=1.0, "Ki"=0.0005}, "L4 PID Gains"={"Kp"=0.1, "Kd"=0.1, "Ki"=0.0005}}, "Stage PID Cluster"={"Stage Z PID"={"Kp"=0.0005, "Kd"=0.001, "Ki"=0.0}, "Stage Y PID"={"Kp"=0.0003, "Kd"=0.01, "Ki"=0.0}, "Stage X PID"={"Kp"=0.0003, "Kd"=0.01, "Ki"=0.0}}, "OCT Z PID Gains"={"Kp"=0.0003, "Kd"=0.0001, "Ki"=0.01}} ("PID Cluster"), "Stage PID Cluster"=w190, "L1 to L4 PID Cluster"=w189, "OCT Z PID Gains"=w188) -> (w187:T12)
            n54 = local read "Offset Home 2 RCM"() -> (w193:dbl[])
            n55 = call "Engaging.vi"("PID Cluster"=w187, "Offset Home 2 RCM"=w193, "error in"=w186, "Engage Pt"=w185, "Prev Posit Cluster"=w184, "FPGA VI Reference In"=w194) -> ("error out"=w183:errorcluster, "Last Posit Cluster"=w192:T14, "FPGA VI Reference Out"=w195:refnum<k20>)  [unwired: 3 in]
          }
          frame "Trajectory Loading" {
            n56 = local read "Offset Home 2 RCM"() -> (w213:dbl[])
            n57 = local read "Stage PID Cluster"() -> (w218:T5)
            n58 = local read "L1 to L4 PID Cluster"() -> (w217:T6)
            n59 = local read "OCT Z PID Gains"() -> (w216:cluster{"Kp":dbl, "Kd":dbl, "Ki":dbl})
            n60 = Bundle By Name(cluster=T12 {"L1 to L4 PID Cluster"={"L1 PID Gains"={"Kp"=0.005, "Kd"=0.5, "Ki"=0.0005}, "L2 PID Gains"={"Kp"=0.01, "Kd"=1.0, "Ki"=0.005}, "L3 PID Gains"={"Kp"=0.05, "Kd"=1.0, "Ki"=0.0005}, "L4 PID Gains"={"Kp"=0.1, "Kd"=0.1, "Ki"=0.0005}}, "Stage PID Cluster"={"Stage Z PID"={"Kp"=0.0005, "Kd"=0.001, "Ki"=0.0}, "Stage Y PID"={"Kp"=0.0003, "Kd"=0.01, "Ki"=0.0}, "Stage X PID"={"Kp"=0.0003, "Kd"=0.01, "Ki"=0.0}}, "OCT Z PID Gains"={"Kp"=0.0003, "Kd"=0.0001, "Ki"=0.01}} ("PID Cluster"), "Stage PID Cluster"=w218, "L1 to L4 PID Cluster"=w217, "OCT Z PID Gains"=w216) -> (w214:T12)
            n61 = call "Trajectory Loading.vi"("PID Cluster"=w214, "error in"=w220, "Offset Home 2 RCM"=w213, "Prev Posit Cluster"=w219, "FPGA VI Reference In"=w221) -> ("Eye Model Cluster"=w200:T4, "Trajectory Cluster"=w196:T2, "Last Posit Cluster"=w206:T14, "FPGA VI Reference Out"=w204:refnum<k20>, "error out"=w210:errorcluster, "First Trk Pt"=→"First Trk Pt":dbl[])  [unwired: 1 in]
            n62 = flat-sequence {
              tunnel: w196 -> [w227]
              tunnel: w200 -> [w228]
              tunnel: w210 -> [w226]
              tunnel: [w226] -> w209
              tunnel: w206 -> [w225]
              tunnel: [w225] -> w205
              tunnel: w204 -> [w224]
              tunnel: [w224] -> w203
              tunnel: [w223] -> w201
              tunnel: w196 -> [w223]
              tunnel: w200 -> [w222]
              tunnel: [w222] -> w199
              tunnel: [w233] -> w208
              tunnel: w209 -> [w233]
              tunnel: [w232] -> w207
              tunnel: w205 -> [w232]
              tunnel: w203 -> [w231]
              tunnel: [w231] -> w202
              tunnel: w201 -> [w230]
              tunnel: w199 -> [w229]
              tunnel: [w230] -> w198
              tunnel: [w229] -> w197
              frame #0 {
                "Eye Model Cluster" <- w228
                "Trajectory Cluster" <- w227
              }
              frame #1 {
                "Update Mdl & Traj" <- TRUE
              }
            }
          }
          frame "Tracking Initialization" {
            n63 = local read "Stage PID Cluster"() -> (w243:T5)
            n64 = local read "L1 to L4 PID Cluster"() -> (w242:T6)
            n65 = local read "OCT Z PID Gains"() -> (w240:cluster{"Kp":dbl, "Kd":dbl, "Ki":dbl})
            n66 = local read "Offset Home 2 RCM"() -> (w244:dbl[])
            n67 = Bundle By Name(cluster=T12 {"L1 to L4 PID Cluster"={"L1 PID Gains"={"Kp"=0.005, "Kd"=0.5, "Ki"=0.0005}, "L2 PID Gains"={"Kp"=0.01, "Kd"=1.0, "Ki"=0.005}, "L3 PID Gains"={"Kp"=0.05, "Kd"=1.0, "Ki"=0.0005}, "L4 PID Gains"={"Kp"=0.1, "Kd"=0.1, "Ki"=0.0005}}, "Stage PID Cluster"={"Stage Z PID"={"Kp"=0.0005, "Kd"=0.001, "Ki"=0.0}, "Stage Y PID"={"Kp"=0.0003, "Kd"=0.01, "Ki"=0.0}, "Stage X PID"={"Kp"=0.0003, "Kd"=0.01, "Ki"=0.0}}, "OCT Z PID Gains"={"Kp"=0.0003, "Kd"=0.0001, "Ki"=0.01}} ("PID Cluster"), "Stage PID Cluster"=w243, "L1 to L4 PID Cluster"=w242, "OCT Z PID Gains"=w240) -> (w239:T12)
            n68 = call "Tracking Initialization.vi"("Eye Model Cluster"=w235, "Trajectory Cluster"=w236, "PID Cluster"=w239, "Offset Home 2 RCM"=w244, "error in"=w249, "Prev Index"=w238, "Prev Posit Cluster"=w245, "FPGA VI Reference In"=w250) -> ("error out"=w247:errorcluster, "Last Index"=w237:i32, "Last Posit Cluster"=w246:T14, "FPGA VI Reference Out"=w248:refnum<k20>)
          }
          frame "Tracking" {
            n69 = local read "Stage PID Cluster"() -> (w260:T5)
            n70 = local read "L1 to L4 PID Cluster"() -> (w259:T6)
            n71 = local read "OCT Z PID Gains"() -> (w258:cluster{"Kp":dbl, "Kd":dbl, "Ki":dbl})
            n72 = local read "Offset Home 2 RCM"() -> (w253:dbl[])
            n73 = Bundle By Name(cluster=T12 {"L1 to L4 PID Cluster"={"L1 PID Gains"={"Kp"=0.005, "Kd"=0.5, "Ki"=0.0005}, "L2 PID Gains"={"Kp"=0.01, "Kd"=1.0, "Ki"=0.005}, "L3 PID Gains"={"Kp"=0.05, "Kd"=1.0, "Ki"=0.0005}, "L4 PID Gains"={"Kp"=0.1, "Kd"=0.1, "Ki"=0.0005}}, "Stage PID Cluster"={"Stage Z PID"={"Kp"=0.0005, "Kd"=0.001, "Ki"=0.0}, "Stage Y PID"={"Kp"=0.0003, "Kd"=0.01, "Ki"=0.0}, "Stage X PID"={"Kp"=0.0003, "Kd"=0.01, "Ki"=0.0}}, "OCT Z PID Gains"={"Kp"=0.0003, "Kd"=0.0001, "Ki"=0.01}} ("PID Cluster"), "Stage PID Cluster"=w260, "L1 to L4 PID Cluster"=w259, "OCT Z PID Gains"=w258) -> (w256:T12)
            n74 = call "Tracking.vi"("Offset Home 2 RCM"=w253, "Trajectory Cluster"=w255, "PID Cluster"=w256, "Eye Model Cluster"=w254, "error in"=w265, "Resume Index"=w252, "Prev Posit Cluster"=w262, "FPGA VI Reference In"=w266) -> ("error out"=w263:errorcluster, "Leave Index"=w251:i32, "Last Posit Cluster"=w261:T14, "FPGA VI Reference Out"=w264:refnum<k20>)
          }
          frame "Rerouting" {
            n75 = local read "Stage PID Cluster"() -> (w279:T5)
            n76 = local read "L1 to L4 PID Cluster"() -> (w278:T6)
            n77 = local read "OCT Z PID Gains"() -> (w277:cluster{"Kp":dbl, "Kd":dbl, "Ki":dbl})
            n78 = local read "Offset Home 2 RCM"() -> (w273:dbl[])
            n79 = Bundle By Name(cluster=T12 {"L1 to L4 PID Cluster"={"L1 PID Gains"={"Kp"=0.005, "Kd"=0.5, "Ki"=0.0005}, "L2 PID Gains"={"Kp"=0.01, "Kd"=1.0, "Ki"=0.005}, "L3 PID Gains"={"Kp"=0.05, "Kd"=1.0, "Ki"=0.0005}, "L4 PID Gains"={"Kp"=0.1, "Kd"=0.1, "Ki"=0.0005}}, "Stage PID Cluster"={"Stage Z PID"={"Kp"=0.0005, "Kd"=0.001, "Ki"=0.0}, "Stage Y PID"={"Kp"=0.0003, "Kd"=0.01, "Ki"=0.0}, "Stage X PID"={"Kp"=0.0003, "Kd"=0.01, "Ki"=0.0}}, "OCT Z PID Gains"={"Kp"=0.0003, "Kd"=0.0001, "Ki"=0.01}} ("PID Cluster"), "Stage PID Cluster"=w279, "L1 to L4 PID Cluster"=w278, "OCT Z PID Gains"=w277) -> (w276:T12)
            n80 = call "Rerouting.vi"("Eye Model Cluster"=w268, "Trajectory Cluster"=w267, "PID Cluster"=w276, "Offset Home 2 RCM"=w273, "error in"=w275, "Prev Index"=w271, "Prev Posit Cluster"=w274, "FPGA VI Reference In"=w281) -> ("error out"=w269:errorcluster, "Last Index"=w270:i32, "Last Posit Cluster"=w272:T14, "FPGA VI Reference Out"=w282:refnum<k20>)
          }
          frame "Regulation" {
            n81 = local read "Engage Pt"() -> (w289:dbl[])
            n82 = local read "Stage PID Cluster"() -> (w297:T5)
            n83 = local read "L1 to L4 PID Cluster"() -> (w296:T6)
            n84 = local read "OCT Z PID Gains"() -> (w295:cluster{"Kp":dbl, "Kd":dbl, "Ki":dbl})
            n85 = Bundle By Name(cluster=T12 {"L1 to L4 PID Cluster"={"L1 PID Gains"={"Kp"=0.005, "Kd"=0.5, "Ki"=0.0005}, "L2 PID Gains"={"Kp"=0.01, "Kd"=1.0, "Ki"=0.005}, "L3 PID Gains"={"Kp"=0.05, "Kd"=1.0, "Ki"=0.0005}, "L4 PID Gains"={"Kp"=0.1, "Kd"=0.1, "Ki"=0.0005}}, "Stage PID Cluster"={"Stage Z PID"={"Kp"=0.0005, "Kd"=0.001, "Ki"=0.0}, "Stage Y PID"={"Kp"=0.0003, "Kd"=0.01, "Ki"=0.0}, "Stage X PID"={"Kp"=0.0003, "Kd"=0.01, "Ki"=0.0}}, "OCT Z PID Gains"={"Kp"=0.0003, "Kd"=0.0001, "Ki"=0.01}} ("PID Cluster"), "Stage PID Cluster"=w297, "L1 to L4 PID Cluster"=w296, "OCT Z PID Gains"=w295) -> (w291:T12)
            n86 = local read "Offset Home 2 RCM"() -> (w294:dbl[])
            n87 = call "Regulation.vi"("PID Cluster"=w291, "Offset Home 2 RCM"=w294, "error in"=w290, "Engage Pt"=w289, "Prev Posit Cluster"=w292, "FPGA VI Reference In"=w293) -> ("error out"=w285:errorcluster, "Last Posit Cluster"=w286:T14, "FPGA VI Reference Out"=w287:refnum<k20>)  [unwired: 3 in]
          }
        }
        n88 = local read "Program Stop"() -> (w110:bool)
      }
      n89 = while {
        shift-right: [w324] -> _
        shift-left: w26 -> [w325]
        shift-right: [w317] -> _
        shift-left: _ -> [w315]
        shift-right: [w316] -> _
        shift-left: _ -> [w314]
        stop <- "Program Stop" stop-if-true
        # "Control and State Logic Loop"
        n90 = Wait (ms)(milliseconds to wait=u32 50) -> ()  [unwired: 1 out]
        n91 = flat-sequence {
          tunnel: [w361] -> w321
          tunnel: [w360] -> w320
          tunnel: w315 -> [w359]
          tunnel: w314 -> [w358]
          tunnel: w321 -> [w389]
          tunnel: w320 -> [w388]
          tunnel: [w389] -> w310
          tunnel: [w388] -> w308
          tunnel: w310 -> [w416]
          tunnel: [w416] -> w309
          tunnel: w308 -> [w433]
          tunnel: [w433] -> w307
          tunnel: [w453] -> w319
          tunnel: w309 -> [w451]
          tunnel: [w451] -> w318
          tunnel: w307 -> [w453]
          tunnel: [w460] -> w316
          tunnel: w319 -> [w460]
          tunnel: [w459] -> w317
          tunnel: w318 -> [w459]
          frame #0 {
            # "Check if Trajectory is (Re)loaded"
            n92 = local read "Update Mdl & Traj"() -> (w363:bool)
            n93 = call "RisingEdge.vi"("Signal In"=w363) -> ("Rising Edge"=w362:bool)  [unwired: 10 in]
            n94 = case shown="True" w362 {
              tunnel: [w364 w385] -> w360
              tunnel: [w365 w374] -> w361
              tunnel: w359 -> [w365 _]
              tunnel: w358 -> [w364 _]
              frame False {
                # "Use Nominal Model & Trajectory"
              }
              frame True {
                w367 = u16 3 items=["4x", "3x", "2x", "1x", "0.5x", "0.2x", "0.1x", "PAUSE"] ("Speed Override")
                w379 = 2 ("index")
                # "Update Trajectory and Model after \"Trajectory Loading\""
                n95 = local read "Trajectory Cluster"() -> (w374:T2)
                n96 = local read "Eye Model Cluster"() -> (w372:T4)
                n97 = local write "Update Mdl & Traj"(FALSE ("Update Model")) -> ()
                n98 = global write "Global Variables.vi" "current run no."(u8 1 ("current run no.")) -> ()
                n99 = local write "Speed Override"(w367) -> ()
                n100 = Unbundle By Name(w374) -> ("Depth Array"=w376:dbl[])
                n101 = shared-variable "PXI-Robot\\JointAngles.lvlib\\Offline Eye Model"(w372) -> ()  [unwired: 1 in, 1 out]
                n102 = call "Extract Depth Param.vi"("Eye Model Cluster"=w372) -> ("Nominal Model param"=w385:T15)
                n103 = Unbundle By Name(w372) -> ("za_true"=w384:dbl, "za_work"=w383:dbl, "zp_work"=→"PO Cruising":dbl, "zp_true"=w381:dbl, "Iris Center"=w378:dbl[])
                n104 = Array Size(array=w376) -> (size(s)=→"No. of Runs":i32)
                n105 = Index Array(array=w378, index=w379) -> (element=w382:dbl)
                n106 = Array Subset(array=w378, index=0, length=w379) -> (w377:dbl[])
                n107 = local write "Iris XY Scaling"(dbl[] [1.0, 1.0]) -> ()
                n108 = local write "Depth Offset"(0.0 ("Depth Offset")) -> ()
                n109 = local write "Rotation"(dbl[] [0.0, 0.0, 0.0]) -> ()
                n110 = local write "PO No-Fly"(w381) -> ()
                n111 = local write "AN No-Fly"(w384) -> ()
                n112 = local write "AN Cruising"(w383) -> ()
                n113 = local write "Iris XY Center"(w377) -> ()
                n114 = local write "Iris Center"(w382) -> ()
              }
            }
          }
          frame #1 {
            # "Update Working Depth After Each Cycle"
            n115 = shared-variable "PXI-Robot\\JointAngles.lvlib\\RemoteSenderEngaged"() -> (w386:bool)  [unwired: 1 in, 1 out]
            n116 = case shown="True" w386 {
              frame False {
                n117 = global write "Global Variables.vi" "assign pt (x,y,z)"("Assign Point [mm]") -> ()
                n118 = global write "Global Variables.vi" "max limit [mmHg]"("Max Limit [mmHg]") -> ()
                n119 = global write "Global Variables.vi" "speed override"("Speed Override") -> ()
              }
              frame True {
                w396 = 2 ("index")
                n120 = disable-structure shown="Disabled" {
                  frame Disabled {
                    n121 = shared-variable "PXI-Robot\\JointAngles.lvlib\\Max Vacuum"() -> (w411:dbl)  [unwired: 1 in, 1 out]
                    n122 = global write "Global Variables.vi" "max limit [mmHg]"(w411) -> ()
                    n123 = local write "Max Limit [mmHg]"(w411) -> ()
                  }
                  frame Enabled {
                  }
                }
                n124 = shared-variable "PXI-Robot\\JointAngles.lvlib\\Assign Point"() -> (w409:dbl[])  [unwired: 1 in, 1 out]
                n125 = shared-variable "PXI-Robot\\JointAngles.lvlib\\EmergencyAlarmBit"() -> (w408:bool)  [unwired: 1 in, 1 out]
                n126 = shared-variable "PXI-Robot\\JointAngles.lvlib\\Go 2 Assign Point"() -> (w405:bool)  [unwired: 1 in, 1 out]
                n127 = shared-variable "PXI-Robot\\JointAngles.lvlib\\Online Eye Model"() -> (w401:T16)  [unwired: 1 in, 1 out]
                n128 = call "RisingEdge.vi"("Signal In"=w405) -> ("Rising Edge"=w406:bool)  [unwired: 10 in]
                n129 = call "RisingEdge.vi"("Signal In"=w408) -> ("Rising Edge"=w407:bool)  [unwired: 10 in]
                n130 = Unbundle By Name(w401) -> ("za_true"=w404:dbl, "za_work"=w403:dbl, "zp_true"=w402:dbl, "Iris Center"=w393:dbl[])
                n131 = global write "Global Variables.vi" "assign pt (x,y,z)"(w409) -> ()
                n132 = local write "Assign Point [mm]"(w409) -> ()
                n133 = local write "Go to Assign Pt"(w406) -> ()
                n134 = case shown="True" w407 {
                  selector: w407 -> [_ w412]
                  frame False {
                  }
                  frame True {
                    n135 = local write "L3 Go Home"(w412) -> ()
                  }
                }
                n136 = Index Array(array=w393, index=w396) -> (element=w394:dbl)
                n137 = Array Subset(array=w393, index=0, length=w396) -> (w397:dbl[])
                n138 = local write "AN No-Fly"(w404) -> ()
                n139 = local write "AN Cruising"(w403) -> ()
                n140 = local write "PO No-Fly"(w402) -> ()
                n141 = local write "Iris XY Center"(w397) -> ()
                n142 = local write "Iris Center"(w394) -> ()
                n143 = shared-variable "PXI-Robot\\JointAngles.lvlib\\Depth Offset"() -> (w400:dbl)  [unwired: 1 in, 1 out]
                n144 = shared-variable "PXI-Robot\\JointAngles.lvlib\\Iris XY Scaling"() -> (w399:dbl[])  [unwired: 1 in, 1 out]
                n145 = shared-variable "PXI-Robot\\JointAngles.lvlib\\DeformArrayRot"() -> (w398:dbl[])  [unwired: 1 in, 1 out]
                n146 = shared-variable "PXI-Robot\\JointAngles.lvlib\\Track Speed"() -> (w410:u16)  [unwired: 1 in, 1 out]
                n147 = global write "Global Variables.vi" "speed override"(w410) -> ()
                n148 = local write "Speed Override"(w410) -> ()
                n149 = local write "Iris XY Scaling"(w399) -> ()
                n150 = local write "Depth Offset"(w400) -> ()
                n151 = local write "Rotation"(w398) -> ()
              }
            }
            n152 = Not(x=w386) -> (.not. x?=w387:bool)
            n153 = global write "Global Variables.vi" "lock robot"(w387) -> ()
          }
          frame #2 {
            n154 = local read "PO No-Fly"() -> (w427:dbl)
            n155 = local read "Iris Center"() -> (w428:dbl)
            n156 = local read "Depth Offset"() -> (w432:dbl)
            n157 = global read "Global Variables.vi" "current run no."() -> (w425:u8)
            n158 = local read "Speed Override"() -> (w422:u16)
            n159 = Unbundle By Name(w416) -> ("Speed Array"=w424:dbl[])
            n160 = Unbundle By Name(w416) -> ("Depth Array"=w423:dbl[])
            n161 = Bundle By Name(cluster=cluster{"zi":dbl, "zp_true":dbl} {"zi"=0.0, "zp_true"=-2.5} ("z Cluster"), "zi"=w428, "zp_true"=w427) -> (w414:cluster{"zi":dbl, "zp_true":dbl})
            n162 = case shown="4" w422 {
              tunnel: [4.0 ("y") 3.0 ("y") 2.0 ("y") 1.0 ("y") 0.5 ("y") 0.2 ("y") 0.1 ("y") 0.0 ("y")] -> w419
              frame 0 {
                # "4X"
              }
              frame 1 {
                # "3X"
              }
              frame 2 {
                # "2X"
              }
              frame 3, Default {
                # "1x"
              }
              frame 4 {
                # "0.5x"
              }
              frame 5 {
                # "0.2x"
              }
              frame 6 {
                # "0.1x"
              }
              frame 7 {
                # "Pause"
              }
            }
            n163 = Increment(x=w425) -> (x+1=w426:u8)
            n164 = call "Depth Control.vi"("Current Run No."=w425, "Depth Offset"=w432, "Depth Array"=w423, "z Cluster"=w414) -> ("zp_work"=w413:dbl, "Schedule Depth & Speed"=w431:cluster{"Next Depth":dbl, "Current Depth":dbl})  [unwired: 6 in]
            n165 = call "Index Param Array.vi"("Index"=w425, "Array Input"=w424) -> ("Index Output"=w420:dbl)  [unwired: 9 in]
            n166 = call "Index Param Array.vi"("Index"=w426, "Array Input"=w424) -> ("Index Output"=w421:dbl)  [unwired: 9 in]
            n167 = Unbundle By Name(w431) -> ("Current Depth"=→"Current Depth":dbl, "Next Depth"=→"Next Depth":dbl)
            n168 = Multiply(x=w421, y=w419) -> (x*y=→"Next Speed":dbl)
            n169 = Multiply(x=w420, y=w419) -> (x*y=→"Current Speed":dbl)
            n170 = local write "PO Cruising"(w413) -> ()
            n171 = shared-variable "PXI-Robot\\JointAngles.lvlib\\PO_cruising"(w413) -> ()  [unwired: 1 in, 1 out]
            n172 = global write "Global Variables.vi" "speed schedule"(w421) -> ()
          }
          frame #3 {
            # "User High-Level Command Override"
            n173 = local read "PO Cruising"() -> (w442:dbl)
            n174 = Bundle By Name(cluster=T1 {"za_true"=0.0, "za_work"=0.0, "zi"=0.0, "zp_work"=0.0, "zp_true"=0.0, "Iris XY Center"=[0.0, 5.0], "Iris XY Scaling"=[1.0, 1.0]} ("High Level cmd"), "za_true"="AN No-Fly", "za_work"="AN Cruising", "zi"="Iris Center", "zp_work"=w442, "zp_true"="PO No-Fly", "Iris XY Center"="Iris XY Center", "Iris XY Scaling"="Iris XY Scaling") -> (w452:T1)
            "Online Eye Model" <- w452
            n175 = call "HighLevelCmdInterpreter.vi"("Nominal Model param"=w453, "High Level cmd"=w452) -> ("Translation Array"=w457:dbl[], "Scaling Array"=w458:dbl[], "PC Displacement"=w454:dbl, "AC Displacement"=w450:dbl)  [unwired: 6 in]
            "Scaling" <- w458
            "Translation" <- w457
            n176 = global write "Global Variables.vi" "PC z displacement"(w454) -> ()
            n177 = global write "Global Variables.vi" "AC z displacement"(w450) -> ()
            n178 = Build Array (concatenate)(w458, "Rotation", w457) -> (w455:dbl[])
            n179 = global write "Global Variables.vi" "deform array"(w455) -> ()
          }
          frame #4 {
            # "Set/Reset Go to Assign Pt Flag"
            n180 = call "RisingEdge.vi"("Signal In"="Go to Assign Pt") -> ("Rising Edge"=w462:bool)  [unwired: 10 in]
            n181 = local write "Go to Assign Pt"(w462) -> ()
          }
        }
        n182 = case shown="\"Regulation\"" w325 {
          selector: w325 -> [w465 w471 w487 w498 w517 w542 w550 w580 w618 w645]
          tunnel: [w464 w472 w486 w497 w518 w543 w551 w581 w619 w646] -> w324
          frame "Homing", Default {
            n183 = global read "Global Variables.vi" "state flag array"() -> (w466:bool[])
            n184 = Index Array(array=w466, index=0) -> (element=w463:bool)
            n185 = case shown="False" w463 {
              tunnel: [w468 w469] -> w464
              tunnel: w465 -> [w468 _]
              frame False {
                # "homing in process"
              }
              frame True {
                w469 = T8."M/S Initialization" ("Current State")
                # "finish homing"
                n186 = global write "Global Variables.vi" "state changing"(TRUE ("state changing")) -> ()
                n187 = local write "Current System State"(w469) -> ()
              }
            }
          }
          frame "M/S Initialization" {
            n188 = global read "Global Variables.vi" "state flag array"() -> (w474:bool[])
            n189 = Index Array(array=w474, index=1) -> (element=w473:bool)
            n190 = case shown="False" w473 {
              tunnel: [w476 w478] -> w472
              tunnel: w471 -> [w476 _]
              frame False {
                n191 = property on="MS/Auto" class="Bool (strict)"("DisabledEnum"=T13."Disabled and Grayed Out" ("Disabled")) -> ()  [unwired: 2 in, 2 out]
              }
              frame True {
                w478 = T8."M/S Operation" ("Current State")
                n192 = global write "Global Variables.vi" "state changing"(TRUE ("state changing")) -> ()
                n193 = property on="MS/Auto" class="Bool (strict)"("DisabledEnum"=T13."Enabled" ("Disabled")) -> ()  [unwired: 2 in, 2 out]
                n194 = local write "Current System State"(w478) -> ()
              }
            }
          }
          frame "M/S Operation" {
            n195 = local read "Load Traj"() -> (w483:bool)
            n196 = local read "MS/Auto"() -> (w485:bool)
            n197 = Not(x=w485) -> (.not. x?=w484:bool)
            n198 = Build Array(w484, w483) -> (w482:bool[])
            n199 = Boolean Array To Number(Boolean array=w482) -> (number=w481:u32)
            n200 = case shown="2" w481 {
              tunnel: w487 -> [w488 _ _]
              tunnel: [w488 w491 w494] -> w486
              frame 0, Default {
              }
              frame 1 {
                w491 = T8."Aiming" ("Current State")
                n201 = global write "Global Variables.vi" "state changing"(TRUE ("state changing")) -> ()
                n202 = property on="MS/Auto" class="Bool (strict)"("DisabledEnum"=T13."Disabled and Grayed Out" ("Disabled")) -> ()  [unwired: 2 in, 2 out]
                n203 = local write "Current System State"(w491) -> ()
              }
              frame 2 {
                w494 = T8."Trajectory Loading" ("Current State")
                n204 = global write "Global Variables.vi" "state changing"(TRUE ("state changing")) -> ()
                n205 = local write "Load Traj"(FALSE ("Load Traj")) -> ()
                n206 = property on="MS/Auto" class="Bool (strict)"("DisabledEnum"=T13."Disabled and Grayed Out" ("Disabled")) -> ()  [unwired: 2 in, 2 out]
                n207 = local write "MS/Auto"(FALSE ("MS/Auto")) -> ()
                n208 = local write "Current System State"(w494) -> ()
              }
            }
          }
          frame "Aiming" {
            n209 = global read "Global Variables.vi" "state flag array"() -> (w500:bool[])
            n210 = Index Array(array=w500, index=3) -> (element=w499:bool)
            n211 = case shown="True" w499 {
              tunnel: w498 -> [w502 w505]
              tunnel: [w502 w504] -> w497
              frame False {
              }
              frame True {
                n212 = property on="MS/Auto" class="Bool (strict)"("DisabledEnum"=T13."Enabled" ("Disabled")) -> ()  [unwired: 2 in, 2 out]
                n213 = Build Array("Insert", "MS/Auto") -> (w509:bool[])
                n214 = Boolean Array To Number(Boolean array=w509) -> (number=w506:u32)
                n215 = case shown="0, Default" w506 {
                  tunnel: w505 -> [w510 _ _]
                  tunnel: [w510 w512 w515] -> w504
                  frame 0, Default {
                  }
                  frame 1 {
                    w512 = T8."Engaging" ("Current State")
                    n216 = global write "Global Variables.vi" "state changing"(TRUE ("state changing")) -> ()
                    n217 = local write "Insert"(FALSE ("Enter")) -> ()
                    n218 = property on="MS/Auto" class="Bool (strict)"("DisabledEnum"=T13."Disabled and Grayed Out" ("Disabled")) -> ()  [unwired: 2 in, 2 out]
                    n219 = local write "Current System State"(w512) -> ()
                  }
                  frame 2 {
                    w515 = T8."M/S Initialization" ("Current State")
                    n220 = global write "Global Variables.vi" "state changing"(TRUE ("state changing")) -> ()
                    n221 = local write "Current System State"(w515) -> ()
                  }
                }
              }
            }
          }
          frame "Engaging" {
            n222 = global read "Global Variables.vi" "state flag array"() -> (w520:bool[])
            n223 = Index Array(array=w520, index=4) -> (element=w519:bool)
            n224 = case shown="True" w519 {
              tunnel: [w523 w530] -> w518
              tunnel: w517 -> [w524 w531]
              frame False {
                n225 = local read "Retract"() -> (w522:bool)
                n226 = case shown="True" w522 {
                  tunnel: [w525 w527] -> w523
                  tunnel: w524 -> [w525 _]
                  frame False {
                  }
                  frame True {
                    w527 = T8."Aiming" ("Current State")
                    n227 = global write "Global Variables.vi" "state changing"(TRUE ("state changing")) -> ()
                    n228 = local write "Retract"(FALSE ("Retract")) -> ()
                    n229 = local write "Current System State"(w527) -> ()
                  }
                }
              }
              frame True {
                n230 = Build Array("Load Traj", "Retract") -> (w534:bool[])
                n231 = Boolean Array To Number(Boolean array=w534) -> (number=w532:u32)
                n232 = case shown="0, Default" w532 {
                  tunnel: w531 -> [w535 _ _]
                  tunnel: [w535 w537 w540] -> w530
                  frame 0, Default {
                  }
                  frame 1 {
                    w537 = T8."Trajectory Loading" ("Current State")
                    n233 = local write "Load Traj"(FALSE ("Load Traj")) -> ()
                    n234 = global write "Global Variables.vi" "state changing"(TRUE ("state changing")) -> ()
                    n235 = local write "Current System State"(w537) -> ()
                  }
                  frame 2 {
                    w540 = T8."Aiming" ("Current State")
                    n236 = global write "Global Variables.vi" "state changing"(TRUE ("state changing")) -> ()
                    n237 = local write "Retract"(FALSE ("Load Traj")) -> ()
                    n238 = local write "Current System State"(w540) -> ()
                  }
                }
              }
            }
          }
          frame "Trajectory Loading" {
            n239 = global read "Global Variables.vi" "state flag array"() -> (w545:bool[])
            n240 = Index Array(array=w545, index=2) -> (element=w544:bool)
            n241 = case shown="False" w544 {
              tunnel: [w547 w548] -> w543
              tunnel: w542 -> [w547 _]
              frame False {
              }
              frame True {
                w548 = T8."Tracking Initialization" ("Current State")
                n242 = global write "Global Variables.vi" "state changing"(TRUE ("state changing")) -> ()
                n243 = local write "Current System State"(w548) -> ()
              }
            }
          }
          frame "Tracking Initialization" {
            n244 = global read "Global Variables.vi" "state flag array"() -> (w553:bool[])
            n245 = Index Array(array=w553, index=5) -> (element=w552:bool)
            n246 = case shown="True" w552 {
              tunnel: [w555 w562] -> w551
              tunnel: w550 -> [w555 w561]
              frame False {
              }
              frame True {
                n247 = local read "Load Traj"() -> (w563:bool)
                n248 = local read "Retract"() -> (w557:bool)
                n249 = local read "To Regulation"() -> (w556:bool)
                n250 = Or(x="Initialize", y=w557) -> (x .or. y?=w559:bool)
                n251 = Build Array("Track", w563, w559, w556) -> (w565:bool[])
                n252 = Boolean Array To Number(Boolean array=w565) -> (number=w564:u32)
                n253 = case shown="4" w564 {
                  tunnel: [w566 w568 w572 w573 w578] -> w562
                  tunnel: w561 -> [w566 _ _ _ _]
                  frame 0, Default {
                  }
                  frame 1 {
                    w568 = T8."Tracking" ("Current State")
                    n254 = global write "Global Variables.vi" "state changing"(TRUE ("state changing")) -> ()
                    n255 = local write "Track"(FALSE ("Track")) -> ()
                    n256 = local write "Current System State"(w568) -> ()
                  }
                  frame 2 {
                    w572 = T8."Trajectory Loading" ("Current State")
                    n257 = global write "Global Variables.vi" "state changing"(TRUE ("state changing")) -> ()
                    n258 = local write "Load Traj"(FALSE ("Load Traj")) -> ()
                    n259 = local write "Current System State"(w572) -> ()
                  }
                  frame 4 {
                    w573 = T8."Engaging" ("Current State")
                    n260 = global write "Global Variables.vi" "state changing"(TRUE ("state changing")) -> ()
                    n261 = local write "Initialize"(FALSE ("Load Traj")) -> ()
                    n262 = local write "Current System State"(w573) -> ()
                  }
                  frame 8 {
                    w576 = FALSE  # Reset
                    w578 = T8."Tracking" ("Current State")
                    n263 = global write "Global Variables.vi" "state changing"(TRUE ("state changing")) -> ()
                    n264 = local write "Track"(FALSE ("Track")) -> ()
                    n265 = local write "Current System State"(w578) -> ()
                    n266 = local write "To Regulation"(w576) -> ()
                  }
                }
              }
            }
          }
          frame "Tracking" {
            n267 = global read "Global Variables.vi" "state flag array"() -> (w583:bool[])
            n268 = Index Array(array=w583, index=6) -> (element=w582:bool)
            n269 = case shown="False" w582 {
              tunnel: [w585 w602] -> w581
              tunnel: w580 -> [w585 w601]
              frame False {
              }
              frame True {
                n270 = local read "Initialize"() -> (w598:bool)
                n271 = local read "Retract"() -> (w595:bool)
                n272 = local read "Go to Assign Pt"() -> (w596:bool)
                n273 = local read "To Regulation"() -> (w597:bool)
                n274 = local read "Timer"() -> (w594:i32)
                n275 = Quotient & Remainder(x=w594, y=90) -> (x-y*floor(x/y)=w592:i32, floor(x/y)=w587:i32)
                n276 = Equal To 0?(x=w592) -> (x = 0?=w591:bool)
                n277 = Not Equal To 0?(x=w587) -> (x != 0?=w586:bool)
                n278 = call "RisingEdge.vi"("Signal In"=w591) -> ("Rising Edge"=w590:bool)  [unwired: 10 in]
                n279 = Compound Arithmetic op=AND(w590, w586, "Stop-and-Go") -> (w589:bool)
                n280 = Build Array(w598, w595, w596, w597, w589) -> (w600:bool[])
                n281 = Boolean Array To Number(Boolean array=w600) -> (number=w599:u32)
                n282 = case shown="16" w599 {
                  tunnel: [w603 w604 w607 w610 w613 w616] -> w602
                  tunnel: w601 -> [w603 _ _ _ _ _]
                  frame 0, Default {
                  }
                  frame 1 {
                    w604 = T8."Engaging" ("Current State")
                    n283 = global write "Global Variables.vi" "state changing"(TRUE ("state changing")) -> ()
                    n284 = local write "Initialize"(FALSE ("Load Traj")) -> ()
                    n285 = local write "Current System State"(w604) -> ()
                  }
                  frame 2 {
                    w607 = T8."Aiming" ("Current State")
                    n286 = global write "Global Variables.vi" "state changing"(TRUE ("state changing")) -> ()
                    n287 = local write "Retract"(FALSE ("Load Traj")) -> ()
                    n288 = local write "Current System State"(w607) -> ()
                  }
                  frame 4 {
                    w610 = T8."Rerouting" ("Current State")
                    n289 = global write "Global Variables.vi" "state changing"(TRUE ("state changing")) -> ()
                    n290 = local write "Go to Assign Pt"(FALSE ("Load Traj")) -> ()
                    n291 = local write "Current System State"(w610) -> ()
                  }
                  frame 8 {
                    w613 = T8."Regulation" ("Current State")
                    n292 = global write "Global Variables.vi" "state changing"(TRUE ("state changing")) -> ()
                    n293 = local write "Current System State"(w613) -> ()
                  }
                  frame 16 {
                    w616 = T8."Regulation" ("Current State")
                    n294 = global write "Global Variables.vi" "state changing"(TRUE ("state changing")) -> ()
                    n295 = local write "To Regulation"(TRUE ("state changing")) -> ()
                    n296 = local write "Current System State"(w616) -> ()
                  }
                }
              }
            }
          }
          frame "Rerouting" {
            n297 = global read "Global Variables.vi" "state flag array"() -> (w621:bool[])
            n298 = Index Array(array=w621, index=7) -> (element=w620:bool)
            n299 = case shown="False" w620 {
              tunnel: [w625 w639] -> w619
              tunnel: w618 -> [w624 _]
              frame False {
                n300 = shared-variable "PXI-Robot\\JointAngles.lvlib\\EmergencyAlarmBit"() -> (w631:bool)  [unwired: 1 in, 1 out]
                n301 = local read "Initialize"() -> (w630:bool)
                n302 = local read "Retract"() -> (w623:bool)
                n303 = local read "Go to Assign Pt"() -> (w627:bool)
                n304 = Compound Arithmetic op=OR(w631, w630, w623) -> (w628:bool)
                n305 = Build Array(w628, w627) -> (w629:bool[])
                n306 = Boolean Array To Number(Boolean array=w629) -> (number=w626:u32)
                n307 = case shown="0, Default" w626 {
                  tunnel: w624 -> [w632 _ _]
                  tunnel: [w632 w633 w636] -> w625
                  frame 0, Default {
                  }
                  frame 1 {
                    w633 = T8."Engaging" ("Current State")
                    n308 = global write "Global Variables.vi" "state changing"(TRUE ("state changing")) -> ()
                    n309 = local write "Initialize"(FALSE ("Initialize")) -> ()
                    n310 = local write "Current System State"(w633) -> ()
                  }
                  frame 2 {
                    w636 = T8."Rerouting" ("Current State")
                    n311 = global write "Global Variables.vi" "state changing"(TRUE ("state changing")) -> ()
                    n312 = local write "Go to Assign Pt"(FALSE ("Initialize")) -> ()
                    n313 = local write "Current System State"(w636) -> ()
                  }
                }
              }
              frame True {
                n314 = local read "To Regulation"() -> (w640:bool)
                n315 = case shown="True" w640 {
                  tunnel: [T8."Tracking" ("Current State") T8."Regulation" ("Current State")] -> w639
                  frame False {
                    n316 = global write "Global Variables.vi" "state changing"(TRUE ("state changing")) -> ()
                  }
                  frame True {
                    n317 = global write "Global Variables.vi" "state changing"(TRUE ("state changing")) -> ()
                  }
                }
                n318 = local write "Current System State"(w639) -> ()
              }
            }
          }
          frame "Regulation" {
            n319 = global read "Global Variables.vi" "state flag array"() -> (w648:bool[])
            n320 = Index Array(array=w648, index=8) -> (element=w647:bool)
            n321 = case shown="True" w647 {
              tunnel: [w657 w669] -> w646
              tunnel: w645 -> [w656 w670]
              frame False {
                n322 = local read "Initialize"() -> (w655:bool)
                n323 = local read "Retract"() -> (w654:bool)
                n324 = local read "Go to Assign Pt"() -> (w650:bool)
                n325 = Or(x=w655, y=w654) -> (x .or. y?=w653:bool)
                n326 = Build Array(w653, w650) -> (w652:bool[])
                n327 = Boolean Array To Number(Boolean array=w652) -> (number=w651:u32)
                n328 = case shown="2" w651 {
                  tunnel: w656 -> [w658 _ _]
                  tunnel: [w658 w660 w663] -> w657
                  frame 0, Default {
                  }
                  frame 1 {
                    w659 = FALSE  # Reset
                    w660 = T8."Engaging" ("Current State")
                    n329 = global write "Global Variables.vi" "state changing"(TRUE ("state changing")) -> ()
                    n330 = local write "Initialize"(FALSE ("Load Traj")) -> ()
                    n331 = local write "Current System State"(w660) -> ()
                    n332 = local write "To Regulation"(w659) -> ()
                  }
                  frame 2 {
                    w663 = T8."Rerouting" ("Current State")
                    n333 = global write "Global Variables.vi" "state changing"(TRUE ("state changing")) -> ()
                    n334 = local write "Go to Assign Pt"(FALSE ("Initialize")) -> ()
                    n335 = local write "Current System State"(w663) -> ()
                  }
                }
              }
              frame True {
                n336 = local read "Load Traj"() -> (w672:bool)
                n337 = local read "Go to Assign Pt"() -> (w673:bool)
                n338 = local read "Initialize"() -> (w668:bool)
                n339 = local read "Retract"() -> (w666:bool)
                n340 = local read "Track"() -> (w667:bool)
                n341 = Build Array(w672, w673, w668, w666, w667) -> (w674:bool[])
                n342 = Boolean Array To Number(Boolean array=w674) -> (number=w671:u32)
                n343 = case shown="2" w671 {
                  tunnel: w670 -> [w675 _ _ _ _ _]
                  tunnel: [w675 w677 w680 w684 w688 w692] -> w669
                  frame 0, Default {
                  }
                  frame 1 {
                    w676 = FALSE  # Reset
                    w677 = T8."Trajectory Loading" ("Current State")
                    n344 = global write "Global Variables.vi" "state changing"(TRUE ("state changing")) -> ()
                    n345 = local write "Load Traj"(FALSE ("Load Traj")) -> ()
                    n346 = local write "To Regulation"(w676) -> ()
                    n347 = local write "Current System State"(w677) -> ()
                  }
                  frame 2 {
                    w680 = T8."Rerouting" ("Current State")
                    n348 = global write "Global Variables.vi" "state changing"(TRUE ("state changing")) -> ()
                    n349 = local write "Go to Assign Pt"(FALSE ("Load Traj")) -> ()
                    n350 = local write "Current System State"(w680) -> ()
                  }
                  frame 4 {
                    w683 = FALSE  # Reset
                    w684 = T8."Engaging" ("Current State")
                    n351 = global write "Global Variables.vi" "state changing"(TRUE ("state changing")) -> ()
                    n352 = local write "Initialize"(FALSE ("Load Traj")) -> ()
                    n353 = local write "To Regulation"(w683) -> ()
                    n354 = local write "Current System State"(w684) -> ()
                  }
                  frame 8 {
                    w687 = FALSE  # Reset
                    w688 = T8."Aiming" ("Current State")
                    n355 = global write "Global Variables.vi" "state changing"(TRUE ("state changing")) -> ()
                    n356 = local write "Retract"(FALSE ("Load Traj")) -> ()
                    n357 = local write "To Regulation"(w687) -> ()
                    n358 = local write "Current System State"(w688) -> ()
                  }
                  frame 16 {
                    w691 = FALSE  # Reset
                    w692 = T8."Tracking" ("Current State")
                    n359 = global write "Global Variables.vi" "state changing"(TRUE ("state changing")) -> ()
                    n360 = local write "Track"(FALSE ("Load Traj")) -> ()
                    n361 = local write "Current System State"(w692) -> ()
                    n362 = local write "To Regulation"(w691) -> ()
                  }
                }
              }
            }
          }
        }
        n363 = Bundle By Name(cluster=T6 {"L1 PID Gains"={"Kp"=0.005, "Kd"=0.5, "Ki"=0.0005}, "L2 PID Gains"={"Kp"=0.01, "Kd"=1.0, "Ki"=0.0005}, "L3 PID Gains"={"Kp"=0.05, "Kd"=1.0, "Ki"=0.0005}, "L4 PID Gains"={"Kp"=0.1, "Kd"=1.0, "Ki"=0.0005}} ("L1 to L4 PID Cluster 2"), "L1 PID Gains"="L1 PID Gains", "L2 PID Gains"="L2 PID Gains", "L3 PID Gains"="L3 PID Gains", "L4 PID Gains"="L4 PID Gains") -> (→"L1 to L4 PID Cluster":T6)
        n364 = Bundle By Name(cluster=T5 {"Stage Z PID"={"Kp"=0.0005, "Kd"=0.001, "Ki"=0.0}, "Stage Y PID"={"Kp"=0.0003, "Kd"=0.01, "Ki"=0.0}, "Stage X PID"={"Kp"=0.0003, "Kd"=0.01, "Ki"=0.0}} ("Stage PID Cluster 2"), "Stage X PID"="Stage X PID Gains", "Stage Y PID"="Stage Y PID Gains", "Stage Z PID"="Stage Z PID Gains") -> (→"Stage PID Cluster":T5)
        n365 = global write "Global Variables.vi" "vac PID gains"("Vac PID Gains") -> ()
        n366 = global write "Global Variables.vi" "increment ctrl"("Inc Ctrl") -> ()
        n367 = global write "Global Variables.vi" "z rot axis"("Z Rot Axis") -> ()
        n368 = global write "Global Variables.vi" "reroute transit vacf"("Reroute Transit Vacf") -> ()
        n369 = global write "Global Variables.vi" "vac extremum"("Vac Extremum") -> ()
        n370 = global write "Global Variables.vi" "z dist thld"("Z Dist Thld") -> ()
        n371 = global write "Global Variables.vi" "joint limits"("Joint Limits") -> ()
        n372 = global write "Global Variables.vi" "refractive index"("Refractice Index") -> ()
        n373 = global write "Global Variables.vi" "min AC gap"("Min AC Gap") -> ()
        n374 = global write "Global Variables.vi" "min PC gap"("Min PC Gap") -> ()
        n375 = global write "Global Variables.vi" "reroute hold [sec]"("Reroute Hold [sec]") -> ()
        n376 = global write "Global Variables.vi" "target IOP"("Target IOP") -> ()
        n377 = global write "Global Variables.vi" "seconds of data"("Seconds of Data") -> ()
        n378 = global write "Global Variables.vi" "L1 to L4 cmd Posit"("Robot Command") -> ()
        n379 = flat-sequence {
          frame #0 {
            n380 = call "RisingEdge.vi"("Signal In"="Take IOP Data") -> ("Rising Edge"=w350:bool)  [unwired: 10 in]
            n381 = case shown="True" w350 {
              selector: w350 -> [_ w352]
              frame False {
              }
              frame True {
                n382 = global write "Global Variables.vi" "take IOP data"(w352) -> ()
              }
            }
          }
          frame #1 {
            n383 = local write "Take IOP Data"(FALSE ("Take IOP Data")) -> ()
          }
        }
        n384 = local read "Program Stop"() -> (w328:bool)
        n385 = Or(x="L3 Go Home", y=w328) -> (x .or. y?=w329:bool)
        n386 = global write "Global Variables.vi" "reset joystick"("Reset Joystick") -> ()
        n387 = global write "Global Variables.vi" "L3 go home"(w329) -> ()
        n388 = global write "Global Variables.vi" "stop accurus"("Stop Accurus") -> ()
        n389 = global write "Global Variables.vi" "go to regulation"("To Regulation") -> ()
        n390 = global write "Global Variables.vi" "vac PID on/off"("PID ON/OFF") -> ()
        n391 = case shown="True" "PID ON/OFF" {
          frame False {
            n392 = global write "Global Variables.vi" "vac cmd"("Vac Cmd") -> ()
            n393 = property on="Vac Cmd" class="DigNum (strict)"("DisabledEnum"=T13."Enabled" ("Disabled")) -> ()  [unwired: 2 in, 2 out]
          }
          frame True {
            n394 = global read "Global Variables.vi" "vac cmd"() -> (w357:sgl)
            n395 = local write "Vac Cmd"(w357) -> ()
            n396 = property on="Vac Cmd" class="DigNum (strict)"("DisabledEnum"=T13."Disabled" ("Disabled")) -> ()  [unwired: 2 in, 2 out]
          }
        }
        n397 = global write "Global Variables.vi" "irrigate"("Irrigation?") -> ()
        n398 = global write "Global Variables.vi" "remote ctrl source"("Remote Control Source") -> ()
        n399 = global write "Global Variables.vi" "vacuum slide"("Control: Vacuum Force") -> ()
        n400 = global write "Global Variables.vi" "program stop"("Program Stop") -> ()
      }
      n401 = while {
        stop <- w82 stop-if-true
        # "Indicator Loop"
        n402 = Wait (ms)(milliseconds to wait=u32 100) -> ()  [unwired: 1 out]
        n403 = global read "Global Variables.vi" "L1 to L4 cmd Posit"() -> (w71:dbl[])
        n404 = global read "Global Variables.vi" "L1 to L4 out Posit"() -> (w74:dbl[])
        n405 = Index Array(array=w74, index #1=0 ("index"), index #2=1 ("index"), index #3=2 ("index"), index #4=3 ("index")) -> (element #1=w77:dbl, element #2=w76:dbl, element #3=w75:dbl, element #4=→"L4 out Posit":dbl)
        "L3 out Posit" <- w75
        "L2 out Posit" <- w76
        "L1 out Posit" <- w77
        n406 = Index Array(array=w71, index #1=0 ("index"), index #2=1 ("index"), index #3=2 ("index"), index #4=3 ("index")) -> (element #1=w81:dbl, element #2=w80:dbl, element #3=w79:dbl, element #4=→"L4 cmd Posit":dbl)
        "L1 cmd Posit" <- w81
        "L3 cmd Posit" <- w79
        "L2 cmd Posit" <- w80
        n407 = call "Forward_Kinematics_v2.vi"("theta 3"=w75, "theta 2"=w76, "theta 1"=w77) -> ("position"=w66:dbl[])
        "Tip out Posit" <- w66
        n408 = call "Forward_Kinematics_v2.vi"("theta 3"=w79, "theta 2"=w80, "theta 1"=w81) -> ("position"=→"Tip cmd Posit":dbl[])
        n409 = shared-variable "PXI-Robot\\JointAngles.lvlib\\ToolTipPosition"(w66) -> ()  [unwired: 1 in, 1 out]
        n410 = global read "Global Variables.vi" "Accurus cluster"() -> (w60:T17)
        n411 = global read "Global Variables.vi" "Stage cmd Posit"() -> (w72:dbl[])
        n412 = global read "Global Variables.vi" "Stage out Posit"() -> (w73:dbl[])
        n413 = Unbundle By Name(w60) -> ("Accurus engaged?"=→"Accurus Engaged?":bool, "Accurus button"=→"Accurus Button":bool[], "Accurus Ch. A Vout"=→"Voltage Output Ch. A":dbl, "Accurus Ch. B Vout"=→"Voltage Output Ch. B":dbl, "Vacuum Force"=→"Vacuum Force [mmHg]" →"Vacuum Force [mmHg]  2":i32, "Irrigation engaged?"=→"Irrigation Engaged?" →"Irrigation Engaged? 2":bool)
        n414 = Index Array(array=w73, index #1=0 ("index"), index #2=1 ("index"), index #3=2 ("index")) -> (element #1=→"X Stage out [mm]" →"X Stage out [mm] 2":dbl, element #2=→"Y Stage out [mm]" →"Y Stage out [mm] 2":dbl, element #3=→"Z Stage out [mm]" →"Z Stage out [mm] 2":dbl)
        n415 = Index Array(array=w72, index #1=0 ("index"), index #2=1 ("index"), index #3=2 ("index")) -> (element #1=→"X Stage cmd [mm]":dbl, element #2=→"Y Stage cmd [mm]":dbl, element #3=→"Z Stage cmd [mm]":dbl)  [unwired: 1 in, 1 out]
        n416 = shared-variable "PXI-Robot\\JointAngles.lvlib\\RemoteSenderEngaged"() -> (→"Remote sender engaged":bool)  [unwired: 1 in, 1 out]
        n417 = shared-variable "PXI-Robot\\JointAngles.lvlib\\EmergencyAlarmBit"() -> (→"Emergency alarm":bool)  [unwired: 1 in, 1 out]
        n418 = global read "Global Variables.vi" "assign pt out of bound"() -> (→"Asgn Pt Out of Bound":bool)
        n419 = global read "Global Variables.vi" "state flag array"() -> (→"State Flag Array":bool[])
        n420 = global read "Global Variables.vi" "state changing"() -> (→"State changing":bool)
        n421 = global read "Global Variables.vi" "file exists?"() -> (→"IOP File Exists":bool)
        n422 = global read "Global Variables.vi" "elapsed time"() -> (→"Elaspsed Time":u16)
        n423 = global read "Global Variables.vi" "OCT Z cmd Posit"() -> (→"OCT Z cmd [mm]":dbl)
        n424 = global read "Global Variables.vi" "OCT Z out Posit"() -> (→"OCT Z out [mm]":dbl)
        n425 = global read "Global Variables.vi" "tracking timer"() -> (w55:i32)
        n426 = global read "Global Variables.vi" "current run no."() -> (→"Current Run No.":u8)
        n427 = global read "Global Variables.vi" "finished late counts"() -> (→"Finished Late Counts":u16)
        n428 = Divide(x=w55, y=10) -> (x/y=→"Timer":dbl)
        n429 = local read "Target IOP"() -> (w43:sgl)
        n430 = local read "Vac Cmd"() -> (w44:sgl)
        n431 = global read "Global Variables.vi" "pressure sensors"() -> (w41:sgl[])
        n432 = local read "Current System State"() -> (w47:T8)
        n433 = Index Array(array=w41, index=2) -> (element=w39:sgl)
        "AC Pressure [mmHg]" <- w39
        n434 = Build Array(w43, w39, w44) -> (w42:sgl[])
        n435 = Array To Cluster(array=w42) -> (cluster=→"IOP Ctrl":T9)
        n436 = shared-variable "PXI-Robot\\JointAngles.lvlib\\SystemState"(w47) -> ()  [unwired: 1 in, 1 out]
        n437 = Array To Cluster(array=w41) -> (cluster=→"Pressure Sensors":T10)
        n438 = case shown="True" "Clear Charts" {
          frame False {
          }
          frame True {
            w103 = T18 [] ("History Data")
            n439 = property on="IOP Ctrl" class="WFChart (strict)"("History Data"=w103) -> ()  [unwired: 2 in, 2 out]
            n440 = property on="Pressure Sensors" class="WFChart (strict)"("History Data"=w103) -> ()  [unwired: 2 in, 2 out]
          }
        }
        n441 = local read "Program Stop"() -> (w82:bool)
      }
      n442 = Build Array(w24, w24, w24, w24, w24, w24, w24, w24) -> (w31:i16[])
      n443 = xnode "Output Shut Down"("FPGA VI Reference In"=w30, "error in"=w29, "AO"=w31, "INHB X"=w32, "INHB Y"=w32, "INHB Z"=w32, "INHB OCT Mot"=w32) -> ("FPGA VI Reference Out"=w27:refnum<k20>, "error out"=w28:errorcluster)
    }
    frame #2 {
      # "Close Applicaion"
      n444 = xnode "FPGA Reset"("FPGA VI Reference In"=w696, "error in"=w695) -> ("FPGA VI Reference Out"=w699:refnum<k20>, "error out"=w698:errorcluster)
      n445 = xnode "Close FPGA VI Reference"("FPGA VI Reference In"=w699, "error in"=w698) -> ("error out"=→"Error(s) Out on Program End":errorcluster)
    }
  }
